vi "cn8202temp_controller.vi"(2 "?":bool, 3 "actions":cluster{bool, bool, bool, bool, bool}, 4 "Holdback (deg C)":dbl min=0.0 max=55.5 format="%.1f", 5 "Ramp Soak Recipe":string[][](table), 6 "Recycle #":dbl min=0.0 max=100.0, 7 "Setpoint (deg C)":dbl max=1200.0 format="%.3f") -> (0 "Current Recipe \nSetpoint (deg C)":dbl format="%.3f", 1 "Thermometer":dbl(slide) scale=0.0..1000.0 scale format="%.2f")   [LabVIEW 2012]
uses:
  <vilib>/Instr/_visa.llb/VISA Configure Serial Port (Instr).vi
panel:
  # "Omega CN8202 Control Program"
  # "Ramp/Soak Parameters"
  # "(0-55.5, 0=off)"
  # "(0-99, 100 = continuous)"
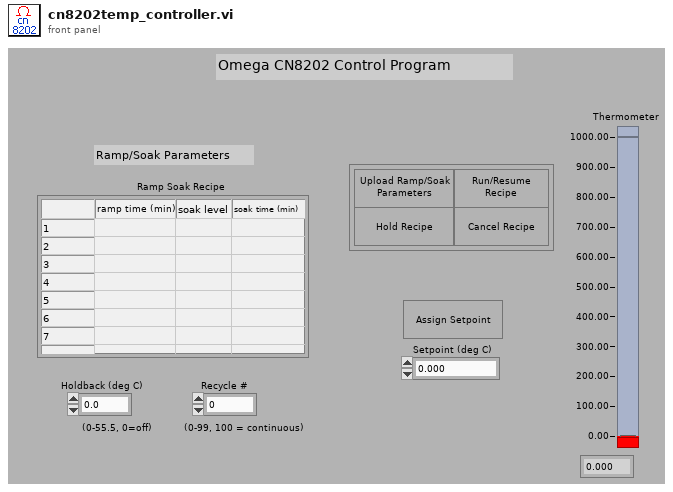
[diagram p1: front panel]
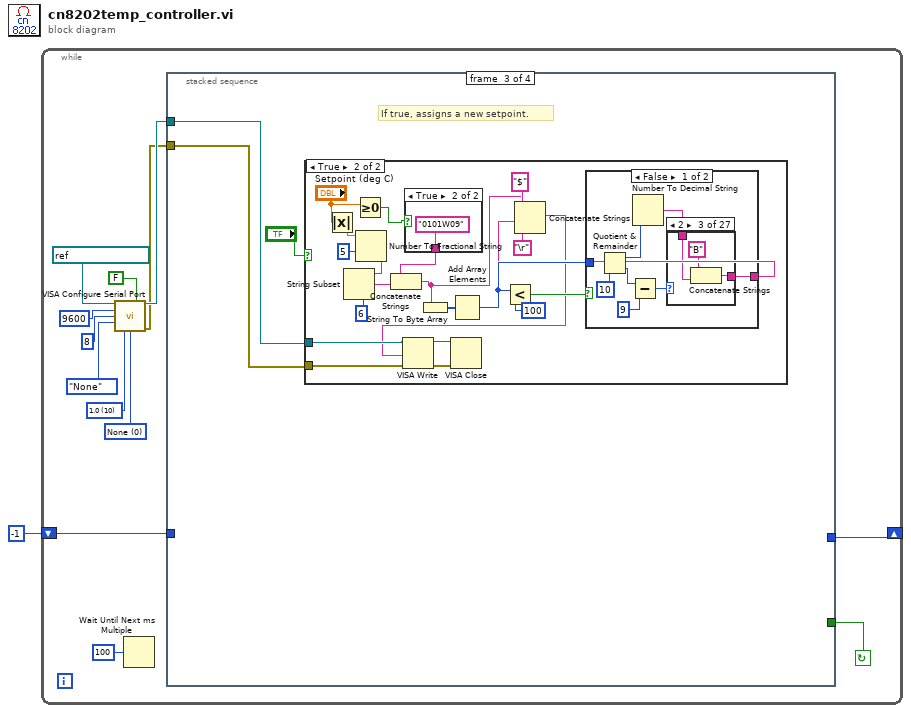
[diagram p0: block diagram]
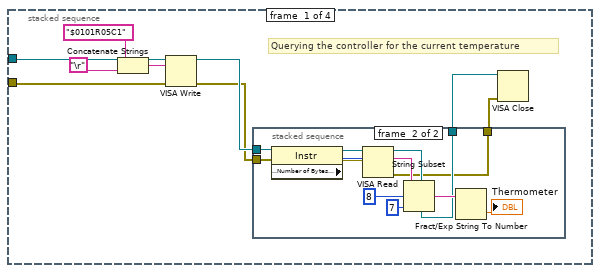
[diagram p2: hidden frame]
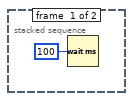
[diagram p3: hidden frame]
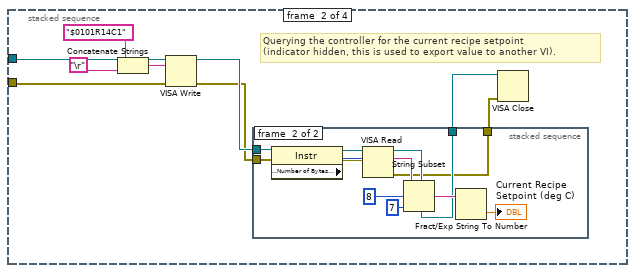
[diagram p4: hidden frame]
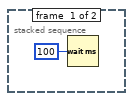
[diagram p5: hidden frame]
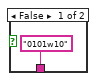
[diagram p7: hidden frame]
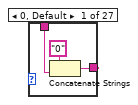
[diagram p8: hidden frame]
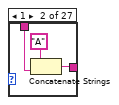
[diagram p9: hidden frame]
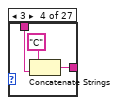
[diagram p10: hidden frame]
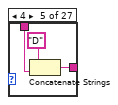
[diagram p11: hidden frame]
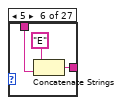
[diagram p12: hidden frame]
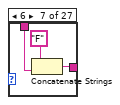
[diagram p13: hidden frame]
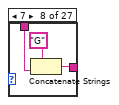
[diagram p14: hidden frame]
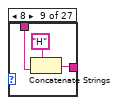
[diagram p15: hidden frame]
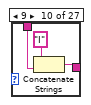
[diagram p16: hidden frame]
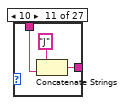
[diagram p17: hidden frame]
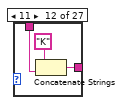
[diagram p18: hidden frame]
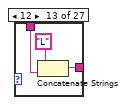
[diagram p19: hidden frame]
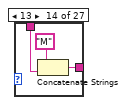
[diagram p20: hidden frame]
diagram:
  n1 = while {
    shift-right: [w2] -> _
    shift-left: -1 -> [w4]
    stop <- w3 continue-if-true
    w11 = u16 0 items=["None"=0, "XON/XOFF"=1, "RTS/CTS"=2, "DTR/DSR"=4] ("flow control (0:none)")
    w12 = u16 10 items=["1.0"=10, "1.5"=15, "2.0"=20] ("stop bits (10: 1 bit)")
    n2 = call-poly "VISA Configure Serial Port"("VISA resource name"=refnum<visa-resource-name> "ASRL1::INSTR", "Enable Termination\nChar (T)"=FALSE ("Enable Termination\nChar (T)"), "baud rate (9600)"=u32 9600, "data bits (8)"=u16 8, "parity (0:none)"=enum16{"None", "Odd", "Even", "Mark", "Space"}."None", "stop bits (10: 1 bit)"=w12, "flow control (0:none)"=w11) -> ("VISA resource name out"=w6:refnum<visa-resource-name>, "error out"=w5:errorcluster)  [unwired: 7 in]
    n3 = Wait Until Next ms Multiple(millisecond multiple=u32 100) -> ()  [unwired: 1 out]
    n4 = stacked-sequence {
      tunnel: w6 -> [w20 w42 w61 w180]
      tunnel: w5 -> [w19 w41 w60 w179]
      tunnel: w4 -> [_ _ _ w178]
      tunnel: [_ _ _ w177] -> w2
      tunnel: [_ _ _ w176] -> w3
      frame #0 {
        # "Querying the controller for the current temperature"
        n5 = Concatenate Strings("$0101R05C1", "\r") -> (w23:string)
        n6 = VISA Write(VISA resource name=w20, write buffer=w23, error in (no error)=w19) -> (VISA resource name out=w18:refnum<visa-resource-name>, error out=w17:errorcluster)  [unwired: 1 out]
        n7 = stacked-sequence {
          tunnel: w18 -> [_ w28]
          tunnel: w17 -> [_ w27]
          tunnel: [_ w26] -> w16
          tunnel: [_ w25] -> w15
          frame #0 {
            n8 = Wait (ms)(milliseconds to wait=u32 100) -> ()  [unwired: 1 out]
          }
          frame #1 {
            n9 = property class="Instr"(reference=w28, error in=w27) -> (reference out=w36:refnum<visa-resource-name>, error out=w34:errorcluster, "Serial Settings:Number of Bytes at Serial Port"=w35:u32)
            n10 = VISA Read(VISA resource name=w36, byte count=w35, error in (no error)=w34) -> (VISA resource name out=w26:refnum<visa-resource-name>, read buffer=w32:string, error out=w25:errorcluster)  [unwired: 1 out]
            n11 = String Subset(string=w32, offset (0)=8, length (rest)=7 ("length (rest)")) -> (substring=w31:string)
            n12 = Fract/Exp String To Number(string=w31) -> (number=→"Thermometer":dbl)  [unwired: 3 in, 1 out]
          }
        }
        n13 = VISA Close(VISA resource name=w16, error in (no error)=w15) -> ()  [unwired: 1 out]
      }
      frame #1 {
        # "Querying the controller for the current recipe setpoint\n(indicator hidden, this is used to export value to another VI)."
        n14 = Concatenate Strings("$0101R14C1", "\r") -> (w45:string)
        n15 = VISA Write(VISA resource name=w42, write buffer=w45, error in (no error)=w41) -> (VISA resource name out=w40:refnum<visa-resource-name>, error out=w39:errorcluster)  [unwired: 1 out]
        n16 = stacked-sequence {
          tunnel: w40 -> [_ w51]
          tunnel: w39 -> [_ w50]
          tunnel: [_ w49] -> w38
          tunnel: [_ w48] -> w37
          frame #0 {
            n17 = Wait (ms)(milliseconds to wait=u32 100) -> ()  [unwired: 1 out]
          }
          frame #1 {
            n18 = property class="Instr"(reference=w51, error in=w50) -> (reference out=w58:refnum<visa-resource-name>, error out=w56:errorcluster, "Serial Settings:Number of Bytes at Serial Port"=w57:u32)
            n19 = VISA Read(VISA resource name=w58, byte count=w57, error in (no error)=w56) -> (VISA resource name out=w49:refnum<visa-resource-name>, read buffer=w54:string, error out=w48:errorcluster)  [unwired: 1 out]
            n20 = String Subset(string=w54, offset (0)=8, length (rest)=7 ("length (rest)")) -> (substring=w53:string)
            n21 = Fract/Exp String To Number(string=w53) -> (number=→"Current Recipe \nSetpoint (deg C)":dbl)  [unwired: 3 in, 1 out]
          }
        }
        n22 = VISA Close(VISA resource name=w38, error in (no error)=w37) -> ()  [unwired: 1 out]
      }
      frame #2 {
        # "If true, assigns a new setpoint."
        n23 = case shown="True" "?" {
          tunnel: w61 -> [_ w66]
          tunnel: w60 -> [_ w65]
          frame False {
          }
          frame True {
            n24 = Absolute Value(x="Setpoint (deg C)") -> (abs(x)=w71:dbl)
            n25 = Greater Or Equal To 0?(x="Setpoint (deg C)") -> (x >= 0?=w72:bool)
            n26 = Number To Fractional String(number=w71, width (-)=i16 5) -> (F-format string=w76:string)  [unwired: 2 in]
            n27 = String Subset(string=w76, length (rest)=6 ("length (rest)")) -> (substring=w73:string)  [unwired: 1 in]
            n28 = case shown="True" w72 {
              tunnel: ["0101w10" "0101W09"] -> w69
              frame False {
              }
              frame True {
              }
            }
            n29 = Concatenate Strings(w69, w73) -> (w62:string)
            n30 = String To Byte Array(string=w62) -> (unsigned byte array=w82:u8[])
            n31 = Add Array Elements(numeric array=w82) -> (sum=w74:u8)
            n32 = Less?(x=w74, y=u8 100) -> (x < y?=w80:bool)
            n33 = case shown="False" w80 {
              tunnel: w74 -> [w88 w175]
              tunnel: [w87 w174] -> w70
              frame False {
                n34 = Quotient & Remainder(x=w88, y=u8 10) -> (x-y*floor(x/y)=w86:u8, floor(x/y)=w89:u8)
                n35 = Subtract(x=w89, y=u8 9) -> (x-y=w91:u8)
                n36 = Number To Decimal String(number=w86) -> (decimal integer string=w92:string)  [unwired: 1 in]
                n37 = case shown="2" w91 {
                  tunnel: w92 -> [w94 w97 w100 w103 w106 w109 w112 w115 w118 w121 w124 w127 w130 w133 w136 w139 w142 w145 w148 w151 w154 w157 w160 w163 w166 w169 w172]
                  tunnel: [w93 w96 w99 w102 w105 w108 w111 w114 w117 w120 w123 w126 w129 w132 w135 w138 w141 w144 w147 w150 w153 w156 w159 w162 w165 w168 w171] -> w87
                  frame 0, Default {
                    n38 = Concatenate Strings("0", w94) -> (w93:string)
                  }
                  frame 1 {
                    n39 = Concatenate Strings("A", w97) -> (w96:string)
                  }
                  frame 2 {
                    n40 = Concatenate Strings("B", w100) -> (w99:string)
                  }
                  frame 3 {
                    n41 = Concatenate Strings("C", w103) -> (w102:string)
                  }
                  frame 4 {
                    n42 = Concatenate Strings("D", w106) -> (w105:string)
                  }
                  frame 5 {
                    n43 = Concatenate Strings("E", w109) -> (w108:string)
                  }
                  frame 6 {
                    n44 = Concatenate Strings("F", w112) -> (w111:string)
                  }
                  frame 7 {
                    n45 = Concatenate Strings("G", w115) -> (w114:string)
                  }
                  frame 8 {
                    n46 = Concatenate Strings("H", w118) -> (w117:string)
                  }
                  frame 9 {
                    n47 = Concatenate Strings("I", w121) -> (w120:string)
                  }
                  frame 10 {
                    n48 = Concatenate Strings("J", w124) -> (w123:string)
                  }
                  frame 11 {
                    n49 = Concatenate Strings("K", w127) -> (w126:string)
                  }
                  frame 12 {
                    n50 = Concatenate Strings("L", w130) -> (w129:string)
                  }
                  frame 13 {
                    n51 = Concatenate Strings("M", w133) -> (w132:string)
                  }
                  frame 14 {
                    n52 = Concatenate Strings("N", w136) -> (w135:string)
                  }
                  frame 15 {
                    n53 = Concatenate Strings("O", w139) -> (w138:string)
                  }
                  frame 16 {
                    n54 = Concatenate Strings("P", w142) -> (w141:string)
                  }
                  frame 17 {
                    n55 = Concatenate Strings("Q", w145) -> (w144:string)
                  }
                  frame 18 {
                    n56 = Concatenate Strings("R", w148) -> (w147:string)
                  }
                  frame 19 {
                    n57 = Concatenate Strings("S", w151) -> (w150:string)
                  }
                  frame 20 {
                    n58 = Concatenate Strings("T", w154) -> (w153:string)
                  }
                  frame 21 {
                    n59 = Concatenate Strings("U", w157) -> (w156:string)
                  }
                  frame 22 {
                    n60 = Concatenate Strings("V", w160) -> (w159:string)
                  }
                  frame 23 {
                    n61 = Concatenate Strings("W", w163) -> (w162:string)
                  }
                  frame 24 {
                    n62 = Concatenate Strings("X", w166) -> (w165:string)
                  }
                  frame 25 {
                    n63 = Concatenate Strings("Y", w169) -> (w168:string)
                  }
                  frame 26 {
                    n64 = Concatenate Strings("Z", w172) -> (w171:string)
                  }
                }
              }
              frame True {
                n65 = Number To Decimal String(number=w175) -> (decimal integer string=w174:string)  [unwired: 1 in]
              }
            }
            n66 = Concatenate Strings("$", w62, w70, "\r") -> (w64:string)
            n67 = VISA Write(VISA resource name=w66, write buffer=w64, error in (no error)=w65) -> (VISA resource name out=w68:refnum<visa-resource-name>, error out=w67:errorcluster)  [unwired: 1 out]
            n68 = VISA Close(VISA resource name=w68, error in (no error)=w67) -> ()  [unwired: 1 out]
          }
        }
      }
      frame #3 {
        n69 = case shown="-1, Default" w178 {
          tunnel: [w181 -1 -1 -1 -1 -1 ("index of element")] -> w177
          tunnel: w180 -> [_ w188 w3077 w3085 w3092 _]
          tunnel: w179 -> [_ w187 w3076 w3086 w3091 _]
          tunnel: [TRUE TRUE TRUE TRUE TRUE FALSE] -> w176
          frame -1, Default {
            # "Check to see which button was pressed\nthen determine which \"state\" to execute next"
            # "No Button Pressed"
            n70 = Cluster To Array(cluster="actions") -> (array=w184:bool[])
            n71 = Search 1D Array(1D array=w184, element=TRUE) -> (index of element=w181:i32)  [unwired: 1 in]
          }
          frame 0 {
            # "Upload Parameters Button Pressed"
            n72 = stacked-sequence {
              tunnel: w188 -> [w192 w2850]
              tunnel: w187 -> [w191 w2849]
              frame #0 {
                # "Set Holdback Button Pressed"
                n73 = for {
                  N: 8 -> [_]
                  tunnel: "Ramp Soak Recipe" -> [w222]
                  tunnel: w192 -> [w201]
                  tunnel: w191 -> [w200]
                  i -> [w221]
                  n74 = Index Array(array=w222, index (row)=w221) -> (element=w220:string[])  [unwired: 1 in]
                  n75 = Index Array(array=w220, index=0) -> (element=w216:string)
                  n76 = Index Array(array=w220, index=1) -> (element=w203:string)
                  n77 = Index Array(array=w220, index=2) -> (element=w204:string)
                  n78 = Fract/Exp String To Number(string=w216) -> (number=w213:dbl)  [unwired: 3 in, 1 out]
                  n79 = Fract/Exp String To Number(string=w203) -> (number=w197:dbl)  [unwired: 3 in, 1 out]
                  n80 = Fract/Exp String To Number(string=w204) -> (number=w206:dbl)  [unwired: 3 in, 1 out]
                  n81 = Absolute Value(x=w197) -> (abs(x)=w194:dbl)
                  n82 = Number To Fractional String(number=w213, width (-)=i16 5) -> (F-format string=w212:string)  [unwired: 2 in]
                  n83 = Number To Fractional String(number=w194, width (-)=i16 5) -> (F-format string=w209:string)  [unwired: 2 in]
                  n84 = Number To Fractional String(number=w206, width (-)=i16 5) -> (F-format string=w205:string)  [unwired: 2 in]
                  n85 = String Subset(string=w212, length (rest)=6 ("length (rest)")) -> (substring=w202:string)  [unwired: 1 in]
                  n86 = String Subset(string=w209, length (rest)=6 ("length (rest)")) -> (substring=w199:string)  [unwired: 1 in]
                  n87 = String Subset(string=w205, length (rest)=6 ("length (rest)")) -> (substring=w198:string)  [unwired: 1 in]
                  n88 = Greater Or Equal To 0?(x=w197) -> (x >= 0?=w196:bool)
                  n89 = case shown="True" w196 {
                    tunnel: ["0101w" "0101W"] -> w195
                    frame False {
                    }
                    frame True {
                    }
                  }
                  n90 = case shown="0, Default" w221 {
                    tunnel: w202 -> [w225 w558 w886 w1214 w1542 w1870 w2198 w2526]
                    tunnel: w201 -> [w229 w556 w884 w1212 w1540 w1868 w2196 w2524]
                    tunnel: w200 -> [w228 w555 w883 w1211 w1539 w1867 w2195 w2523]
                    tunnel: w199 -> [w230 w557 w885 w1213 w1541 w1869 w2197 w2525]
                    tunnel: w198 -> [w227 w554 w882 w1210 w1538 w1866 w2194 w2522]
                    tunnel: w195 -> [w226 w553 w881 w1209 w1537 w1865 w2193 w2521]
                    frame 0, Default {
                      n91 = stacked-sequence {
                        tunnel: w225 -> [w239 _ _]
                        tunnel: w230 -> [_ w340 _]
                        tunnel: w229 -> [w233 w344 w450]
                        tunnel: w228 -> [w232 w343 w449]
                        tunnel: w227 -> [_ _ w447]
                        tunnel: w226 -> [_ w338 _]
                        frame #0 {
                          n92 = Wait Until Next ms Multiple(millisecond multiple=u32 300) -> ()  [unwired: 1 out]
                          n93 = Concatenate Strings("0101W42", w239) -> (w241:string)
                          n94 = String To Byte Array(string=w241) -> (unsigned byte array=w245:u8[])
                          n95 = Add Array Elements(numeric array=w245) -> (sum=w236:u8)
                          n96 = Less?(x=w236, y=u8 100) -> (x < y?=w238:bool)
                          n97 = case shown="False" w238 {
                            tunnel: w236 -> [w250 w337]
                            tunnel: [w249 w336] -> w237
                            frame False {
                              n98 = Quotient & Remainder(x=w250, y=u8 10) -> (x-y*floor(x/y)=w248:u8, floor(x/y)=w251:u8)
                              n99 = Subtract(x=w251, y=u8 9) -> (x-y=w253:u8)
                              n100 = Number To Decimal String(number=w248) -> (decimal integer string=w254:string)  [unwired: 1 in]
                              n101 = case shown="6" w253 {
                                tunnel: w254 -> [w256 w259 w262 w265 w268 w271 w274 w277 w280 w283 w286 w289 w292 w295 w298 w301 w304 w307 w310 w313 w316 w319 w322 w325 w328 w331 w334]
                                tunnel: [w255 w258 w261 w264 w267 w270 w273 w276 w279 w282 w285 w288 w291 w294 w297 w300 w303 w306 w309 w312 w315 w318 w321 w324 w327 w330 w333] -> w249
                                frame 0, Default {
                                n102 = Concatenate Strings("0", w256) -> (w255:string)
                                }
                                frame 1 {
                                n103 = Concatenate Strings("A", w259) -> (w258:string)
                                }
                                frame 2 {
                                n104 = Concatenate Strings("B", w262) -> (w261:string)
                                }
                                frame 3 {
                                n105 = Concatenate Strings("C", w265) -> (w264:string)
                                }
                                frame 4 {
                                n106 = Concatenate Strings("D", w268) -> (w267:string)
                                }
                                frame 5 {
                                n107 = Concatenate Strings("E", w271) -> (w270:string)
                                }
                                frame 6 {
                                n108 = Concatenate Strings("F", w274) -> (w273:string)
                                }
                                frame 7 {
                                n109 = Concatenate Strings("G", w277) -> (w276:string)
                                }
                                frame 8 {
                                n110 = Concatenate Strings("H", w280) -> (w279:string)
                                }
                                frame 9 {
                                n111 = Concatenate Strings("I", w283) -> (w282:string)
                                }
                                frame 10 {
                                n112 = Concatenate Strings("J", w286) -> (w285:string)
                                }
                                frame 11 {
                                n113 = Concatenate Strings("K", w289) -> (w288:string)
                                }
                                frame 12 {
                                n114 = Concatenate Strings("L", w292) -> (w291:string)
                                }
                                frame 13 {
                                n115 = Concatenate Strings("M", w295) -> (w294:string)
                                }
                                frame 14 {
                                n116 = Concatenate Strings("N", w298) -> (w297:string)
                                }
                                frame 15 {
                                n117 = Concatenate Strings("O", w301) -> (w300:string)
                                }
                                frame 16 {
                                n118 = Concatenate Strings("P", w304) -> (w303:string)
                                }
                                frame 17 {
                                n119 = Concatenate Strings("Q", w307) -> (w306:string)
                                }
                                frame 18 {
                                n120 = Concatenate Strings("R", w310) -> (w309:string)
                                }
                                frame 19 {
                                n121 = Concatenate Strings("S", w313) -> (w312:string)
                                }
                                frame 20 {
                                n122 = Concatenate Strings("T", w316) -> (w315:string)
                                }
                                frame 21 {
                                n123 = Concatenate Strings("U", w319) -> (w318:string)
                                }
                                frame 22 {
                                n124 = Concatenate Strings("V", w322) -> (w321:string)
                                }
                                frame 23 {
                                n125 = Concatenate Strings("W", w325) -> (w324:string)
                                }
                                frame 24 {
                                n126 = Concatenate Strings("X", w328) -> (w327:string)
                                }
                                frame 25 {
                                n127 = Concatenate Strings("Y", w331) -> (w330:string)
                                }
                                frame 26 {
                                n128 = Concatenate Strings("Z", w334) -> (w333:string)
                                }
                              }
                            }
                            frame True {
                              n129 = Number To Decimal String(number=w337) -> (decimal integer string=w336:string)  [unwired: 1 in]
                            }
                          }
                          n130 = Concatenate Strings("$", w241, w237, "\r") -> (w246:string)
                          n131 = VISA Write(VISA resource name=w233, write buffer=w246, error in (no error)=w232) -> (VISA resource name out=w235:refnum<visa-resource-name>, error out=w234:errorcluster)  [unwired: 1 out]
                          n132 = VISA Close(VISA resource name=w235, error in (no error)=w234) -> ()  [unwired: 1 out]
                        }
                        frame #1 {
                          n133 = Wait Until Next ms Multiple(millisecond multiple=u32 300) -> ()  [unwired: 1 out]
                          n134 = Concatenate Strings(w338, "58", w340) -> (w350:string)
                          n135 = String To Byte Array(string=w350) -> (unsigned byte array=w354:u8[])
                          n136 = Add Array Elements(numeric array=w354) -> (sum=w347:u8)
                          n137 = Less?(x=w347, y=u8 100) -> (x < y?=w349:bool)
                          n138 = case shown="False" w349 {
                            tunnel: w347 -> [w358 w445]
                            tunnel: [w357 w444] -> w348
                            frame False {
                              n139 = Quotient & Remainder(x=w358, y=u8 10) -> (x-y*floor(x/y)=w356:u8, floor(x/y)=w359:u8)
                              n140 = Subtract(x=w359, y=u8 9) -> (x-y=w361:u8)
                              n141 = Number To Decimal String(number=w356) -> (decimal integer string=w362:string)  [unwired: 1 in]
                              n142 = case shown="7" w361 {
                                tunnel: w362 -> [w364 w367 w370 w373 w376 w379 w382 w385 w388 w391 w394 w397 w400 w403 w406 w409 w412 w415 w418 w421 w424 w427 w430 w433 w436 w439 w442]
                                tunnel: [w363 w366 w369 w372 w375 w378 w381 w384 w387 w390 w393 w396 w399 w402 w405 w408 w411 w414 w417 w420 w423 w426 w429 w432 w435 w438 w441] -> w357
                                frame 0, Default {
                                n143 = Concatenate Strings("0", w364) -> (w363:string)
                                }
                                frame 1 {
                                n144 = Concatenate Strings("A", w367) -> (w366:string)
                                }
                                frame 2 {
                                n145 = Concatenate Strings("B", w370) -> (w369:string)
                                }
                                frame 3 {
                                n146 = Concatenate Strings("C", w373) -> (w372:string)
                                }
                                frame 4 {
                                n147 = Concatenate Strings("D", w376) -> (w375:string)
                                }
                                frame 5 {
                                n148 = Concatenate Strings("E", w379) -> (w378:string)
                                }
                                frame 6 {
                                n149 = Concatenate Strings("F", w382) -> (w381:string)
                                }
                                frame 7 {
                                n150 = Concatenate Strings("G", w385) -> (w384:string)
                                }
                                frame 8 {
                                n151 = Concatenate Strings("H", w388) -> (w387:string)
                                }
                                frame 9 {
                                n152 = Concatenate Strings("I", w391) -> (w390:string)
                                }
                                frame 10 {
                                n153 = Concatenate Strings("J", w394) -> (w393:string)
                                }
                                frame 11 {
                                n154 = Concatenate Strings("K", w397) -> (w396:string)
                                }
                                frame 12 {
                                n155 = Concatenate Strings("L", w400) -> (w399:string)
                                }
                                frame 13 {
                                n156 = Concatenate Strings("M", w403) -> (w402:string)
                                }
                                frame 14 {
                                n157 = Concatenate Strings("N", w406) -> (w405:string)
                                }
                                frame 15 {
                                n158 = Concatenate Strings("O", w409) -> (w408:string)
                                }
                                frame 16 {
                                n159 = Concatenate Strings("P", w412) -> (w411:string)
                                }
                                frame 17 {
                                n160 = Concatenate Strings("Q", w415) -> (w414:string)
                                }
                                frame 18 {
                                n161 = Concatenate Strings("R", w418) -> (w417:string)
                                }
                                frame 19 {
                                n162 = Concatenate Strings("S", w421) -> (w420:string)
                                }
                                frame 20 {
                                n163 = Concatenate Strings("T", w424) -> (w423:string)
                                }
                                frame 21 {
                                n164 = Concatenate Strings("U", w427) -> (w426:string)
                                }
                                frame 22 {
                                n165 = Concatenate Strings("V", w430) -> (w429:string)
                                }
                                frame 23 {
                                n166 = Concatenate Strings("W", w433) -> (w432:string)
                                }
                                frame 24 {
                                n167 = Concatenate Strings("X", w436) -> (w435:string)
                                }
                                frame 25 {
                                n168 = Concatenate Strings("Y", w439) -> (w438:string)
                                }
                                frame 26 {
                                n169 = Concatenate Strings("Z", w442) -> (w441:string)
                                }
                              }
                            }
                            frame True {
                              n170 = Number To Decimal String(number=w445) -> (decimal integer string=w444:string)  [unwired: 1 in]
                            }
                          }
                          n171 = Concatenate Strings("$", w350, w348, "\r") -> (w342:string)
                          n172 = VISA Write(VISA resource name=w344, write buffer=w342, error in (no error)=w343) -> (VISA resource name out=w346:refnum<visa-resource-name>, error out=w345:errorcluster)  [unwired: 1 out]
                          n173 = VISA Close(VISA resource name=w346, error in (no error)=w345) -> ()  [unwired: 1 out]
                        }
                        frame #2 {
                          n174 = Wait Until Next ms Multiple(millisecond multiple=u32 300) -> ()  [unwired: 1 out]
                          n175 = Concatenate Strings("0101W66", w447) -> (w457:string)
                          n176 = String To Byte Array(string=w457) -> (unsigned byte array=w461:u8[])
                          n177 = Add Array Elements(numeric array=w461) -> (sum=w453:u8)
                          n178 = Less?(x=w453, y=u8 100) -> (x < y?=w455:bool)
                          n179 = case shown="False" w455 {
                            tunnel: w453 -> [w465 w552]
                            tunnel: [w464 w551] -> w454
                            frame False {
                              n180 = Quotient & Remainder(x=w465, y=u8 10) -> (x-y*floor(x/y)=w463:u8, floor(x/y)=w466:u8)
                              n181 = Subtract(x=w466, y=u8 9) -> (x-y=w468:u8)
                              n182 = Number To Decimal String(number=w463) -> (decimal integer string=w469:string)  [unwired: 1 in]
                              n183 = case shown="7" w468 {
                                tunnel: w469 -> [w471 w474 w477 w480 w483 w486 w489 w492 w495 w498 w501 w504 w507 w510 w513 w516 w519 w522 w525 w528 w531 w534 w537 w540 w543 w546 w549]
                                tunnel: [w470 w473 w476 w479 w482 w485 w488 w491 w494 w497 w500 w503 w506 w509 w512 w515 w518 w521 w524 w527 w530 w533 w536 w539 w542 w545 w548] -> w464
                                frame 0, Default {
                                n184 = Concatenate Strings("0", w471) -> (w470:string)
                                }
                                frame 1 {
                                n185 = Concatenate Strings("A", w474) -> (w473:string)
                                }
                                frame 2 {
                                n186 = Concatenate Strings("B", w477) -> (w476:string)
                                }
                                frame 3 {
                                n187 = Concatenate Strings("C", w480) -> (w479:string)
                                }
                                frame 4 {
                                n188 = Concatenate Strings("D", w483) -> (w482:string)
                                }
                                frame 5 {
                                n189 = Concatenate Strings("E", w486) -> (w485:string)
                                }
                                frame 6 {
                                n190 = Concatenate Strings("F", w489) -> (w488:string)
                                }
                                frame 7 {
                                n191 = Concatenate Strings("G", w492) -> (w491:string)
                                }
                                frame 8 {
                                n192 = Concatenate Strings("H", w495) -> (w494:string)
                                }
                                frame 9 {
                                n193 = Concatenate Strings("I", w498) -> (w497:string)
                                }
                                frame 10 {
                                n194 = Concatenate Strings("J", w501) -> (w500:string)
                                }
                                frame 11 {
                                n195 = Concatenate Strings("K", w504) -> (w503:string)
                                }
                                frame 12 {
                                n196 = Concatenate Strings("L", w507) -> (w506:string)
                                }
                                frame 13 {
                                n197 = Concatenate Strings("M", w510) -> (w509:string)
                                }
                                frame 14 {
                                n198 = Concatenate Strings("N", w513) -> (w512:string)
                                }
                                frame 15 {
                                n199 = Concatenate Strings("O", w516) -> (w515:string)
                                }
                                frame 16 {
                                n200 = Concatenate Strings("P", w519) -> (w518:string)
                                }
                                frame 17 {
                                n201 = Concatenate Strings("Q", w522) -> (w521:string)
                                }
                                frame 18 {
                                n202 = Concatenate Strings("R", w525) -> (w524:string)
                                }
                                frame 19 {
                                n203 = Concatenate Strings("S", w528) -> (w527:string)
                                }
                                frame 20 {
                                n204 = Concatenate Strings("T", w531) -> (w530:string)
                                }
                                frame 21 {
                                n205 = Concatenate Strings("U", w534) -> (w533:string)
                                }
                                frame 22 {
                                n206 = Concatenate Strings("V", w537) -> (w536:string)
                                }
                                frame 23 {
                                n207 = Concatenate Strings("W", w540) -> (w539:string)
                                }
                                frame 24 {
                                n208 = Concatenate Strings("X", w543) -> (w542:string)
                                }
                                frame 25 {
                                n209 = Concatenate Strings("Y", w546) -> (w545:string)
                                }
                                frame 26 {
                                n210 = Concatenate Strings("Z", w549) -> (w548:string)
                                }
                              }
                            }
                            frame True {
                              n211 = Number To Decimal String(number=w552) -> (decimal integer string=w551:string)  [unwired: 1 in]
                            }
                          }
                          n212 = Concatenate Strings("$", w457, w454, "\r") -> (w448:string)
                          n213 = VISA Write(VISA resource name=w450, write buffer=w448, error in (no error)=w449) -> (VISA resource name out=w452:refnum<visa-resource-name>, error out=w451:errorcluster)  [unwired: 1 out]
                          n214 = VISA Close(VISA resource name=w452, error in (no error)=w451) -> ()  [unwired: 1 out]
                        }
                      }
                    }
                    frame 1 {
                      n215 = stacked-sequence {
                        tunnel: w558 -> [w567 _ _]
                        tunnel: w557 -> [_ w668 _]
                        tunnel: w556 -> [w561 w672 w778]
                        tunnel: w555 -> [w560 w671 w777]
                        tunnel: w554 -> [_ _ w775]
                        tunnel: w553 -> [_ w666 _]
                        frame #0 {
                          n216 = Wait Until Next ms Multiple(millisecond multiple=u32 300) -> ()  [unwired: 1 out]
                          n217 = Concatenate Strings("0101W43", w567) -> (w569:string)
                          n218 = String To Byte Array(string=w569) -> (unsigned byte array=w573:u8[])
                          n219 = Add Array Elements(numeric array=w573) -> (sum=w564:u8)
                          n220 = Less?(x=w564, y=u8 100) -> (x < y?=w566:bool)
                          n221 = case shown="False" w566 {
                            tunnel: w564 -> [w578 w665]
                            tunnel: [w577 w664] -> w565
                            frame False {
                              n222 = Quotient & Remainder(x=w578, y=u8 10) -> (x-y*floor(x/y)=w576:u8, floor(x/y)=w579:u8)
                              n223 = Subtract(x=w579, y=u8 9) -> (x-y=w581:u8)
                              n224 = Number To Decimal String(number=w576) -> (decimal integer string=w582:string)  [unwired: 1 in]
                              n225 = case shown="8" w581 {
                                tunnel: w582 -> [w584 w587 w590 w593 w596 w599 w602 w605 w608 w611 w614 w617 w620 w623 w626 w629 w632 w635 w638 w641 w644 w647 w650 w653 w656 w659 w662]
                                tunnel: [w583 w586 w589 w592 w595 w598 w601 w604 w607 w610 w613 w616 w619 w622 w625 w628 w631 w634 w637 w640 w643 w646 w649 w652 w655 w658 w661] -> w577
                                frame 0, Default {
                                n226 = Concatenate Strings("0", w584) -> (w583:string)
                                }
                                frame 1 {
                                n227 = Concatenate Strings("A", w587) -> (w586:string)
                                }
                                frame 2 {
                                n228 = Concatenate Strings("B", w590) -> (w589:string)
                                }
                                frame 3 {
                                n229 = Concatenate Strings("C", w593) -> (w592:string)
                                }
                                frame 4 {
                                n230 = Concatenate Strings("D", w596) -> (w595:string)
                                }
                                frame 5 {
                                n231 = Concatenate Strings("E", w599) -> (w598:string)
                                }
                                frame 6 {
                                n232 = Concatenate Strings("F", w602) -> (w601:string)
                                }
                                frame 7 {
                                n233 = Concatenate Strings("G", w605) -> (w604:string)
                                }
                                frame 8 {
                                n234 = Concatenate Strings("H", w608) -> (w607:string)
                                }
                                frame 9 {
                                n235 = Concatenate Strings("I", w611) -> (w610:string)
                                }
                                frame 10 {
                                n236 = Concatenate Strings("J", w614) -> (w613:string)
                                }
                                frame 11 {
                                n237 = Concatenate Strings("K", w617) -> (w616:string)
                                }
                                frame 12 {
                                n238 = Concatenate Strings("L", w620) -> (w619:string)
                                }
                                frame 13 {
                                n239 = Concatenate Strings("M", w623) -> (w622:string)
                                }
                                frame 14 {
                                n240 = Concatenate Strings("N", w626) -> (w625:string)
                                }
                                frame 15 {
                                n241 = Concatenate Strings("O", w629) -> (w628:string)
                                }
                                frame 16 {
                                n242 = Concatenate Strings("P", w632) -> (w631:string)
                                }
                                frame 17 {
                                n243 = Concatenate Strings("Q", w635) -> (w634:string)
                                }
                                frame 18 {
                                n244 = Concatenate Strings("R", w638) -> (w637:string)
                                }
                                frame 19 {
                                n245 = Concatenate Strings("S", w641) -> (w640:string)
                                }
                                frame 20 {
                                n246 = Concatenate Strings("T", w644) -> (w643:string)
                                }
                                frame 21 {
                                n247 = Concatenate Strings("U", w647) -> (w646:string)
                                }
                                frame 22 {
                                n248 = Concatenate Strings("V", w650) -> (w649:string)
                                }
                                frame 23 {
                                n249 = Concatenate Strings("W", w653) -> (w652:string)
                                }
                                frame 24 {
                                n250 = Concatenate Strings("X", w656) -> (w655:string)
                                }
                                frame 25 {
                                n251 = Concatenate Strings("Y", w659) -> (w658:string)
                                }
                                frame 26 {
                                n252 = Concatenate Strings("Z", w662) -> (w661:string)
                                }
                              }
                            }
                            frame True {
                              n253 = Number To Decimal String(number=w665) -> (decimal integer string=w664:string)  [unwired: 1 in]
                            }
                          }
                          n254 = Concatenate Strings("$", w569, w565, "\r") -> (w574:string)
                          n255 = VISA Write(VISA resource name=w561, write buffer=w574, error in (no error)=w560) -> (VISA resource name out=w563:refnum<visa-resource-name>, error out=w562:errorcluster)  [unwired: 1 out]
                          n256 = VISA Close(VISA resource name=w563, error in (no error)=w562) -> ()  [unwired: 1 out]
                        }
                        frame #1 {
                          n257 = Wait Until Next ms Multiple(millisecond multiple=u32 300) -> ()  [unwired: 1 out]
                          n258 = Concatenate Strings(w666, "59", w668) -> (w678:string)
                          n259 = String To Byte Array(string=w678) -> (unsigned byte array=w682:u8[])
                          n260 = Add Array Elements(numeric array=w682) -> (sum=w675:u8)
                          n261 = Less?(x=w675, y=u8 100) -> (x < y?=w677:bool)
                          n262 = case shown="False" w677 {
                            tunnel: w675 -> [w686 w773]
                            tunnel: [w685 w772] -> w676
                            frame False {
                              n263 = Quotient & Remainder(x=w686, y=u8 10) -> (x-y*floor(x/y)=w684:u8, floor(x/y)=w687:u8)
                              n264 = Subtract(x=w687, y=u8 9) -> (x-y=w689:u8)
                              n265 = Number To Decimal String(number=w684) -> (decimal integer string=w690:string)  [unwired: 1 in]
                              n266 = case shown="10" w689 {
                                tunnel: w690 -> [w692 w695 w698 w701 w704 w707 w710 w713 w716 w719 w722 w725 w728 w731 w734 w737 w740 w743 w746 w749 w752 w755 w758 w761 w764 w767 w770]
                                tunnel: [w691 w694 w697 w700 w703 w706 w709 w712 w715 w718 w721 w724 w727 w730 w733 w736 w739 w742 w745 w748 w751 w754 w757 w760 w763 w766 w769] -> w685
                                frame 0, Default {
                                n267 = Concatenate Strings("0", w692) -> (w691:string)
                                }
                                frame 1 {
                                n268 = Concatenate Strings("A", w695) -> (w694:string)
                                }
                                frame 2 {
                                n269 = Concatenate Strings("B", w698) -> (w697:string)
                                }
                                frame 3 {
                                n270 = Concatenate Strings("C", w701) -> (w700:string)
                                }
                                frame 4 {
                                n271 = Concatenate Strings("D", w704) -> (w703:string)
                                }
                                frame 5 {
                                n272 = Concatenate Strings("E", w707) -> (w706:string)
                                }
                                frame 6 {
                                n273 = Concatenate Strings("F", w710) -> (w709:string)
                                }
                                frame 7 {
                                n274 = Concatenate Strings("G", w713) -> (w712:string)
                                }
                                frame 8 {
                                n275 = Concatenate Strings("H", w716) -> (w715:string)
                                }
                                frame 9 {
                                n276 = Concatenate Strings("I", w719) -> (w718:string)
                                }
                                frame 10 {
                                n277 = Concatenate Strings("J", w722) -> (w721:string)
                                }
                                frame 11 {
                                n278 = Concatenate Strings("K", w725) -> (w724:string)
                                }
                                frame 12 {
                                n279 = Concatenate Strings("L", w728) -> (w727:string)
                                }
                                frame 13 {
                                n280 = Concatenate Strings("M", w731) -> (w730:string)
                                }
                                frame 14 {
                                n281 = Concatenate Strings("N", w734) -> (w733:string)
                                }
                                frame 15 {
                                n282 = Concatenate Strings("O", w737) -> (w736:string)
                                }
                                frame 16 {
                                n283 = Concatenate Strings("P", w740) -> (w739:string)
                                }
                                frame 17 {
                                n284 = Concatenate Strings("Q", w743) -> (w742:string)
                                }
                                frame 18 {
                                n285 = Concatenate Strings("R", w746) -> (w745:string)
                                }
                                frame 19 {
                                n286 = Concatenate Strings("S", w749) -> (w748:string)
                                }
                                frame 20 {
                                n287 = Concatenate Strings("T", w752) -> (w751:string)
                                }
                                frame 21 {
                                n288 = Concatenate Strings("U", w755) -> (w754:string)
                                }
                                frame 22 {
                                n289 = Concatenate Strings("V", w758) -> (w757:string)
                                }
                                frame 23 {
                                n290 = Concatenate Strings("W", w761) -> (w760:string)
                                }
                                frame 24 {
                                n291 = Concatenate Strings("X", w764) -> (w763:string)
                                }
                                frame 25 {
                                n292 = Concatenate Strings("Y", w767) -> (w766:string)
                                }
                                frame 26 {
                                n293 = Concatenate Strings("Z", w770) -> (w769:string)
                                }
                              }
                            }
                            frame True {
                              n294 = Number To Decimal String(number=w773) -> (decimal integer string=w772:string)  [unwired: 1 in]
                            }
                          }
                          n295 = Concatenate Strings("$", w678, w676, "\r") -> (w670:string)
                          n296 = VISA Write(VISA resource name=w672, write buffer=w670, error in (no error)=w671) -> (VISA resource name out=w674:refnum<visa-resource-name>, error out=w673:errorcluster)  [unwired: 1 out]
                          n297 = VISA Close(VISA resource name=w674, error in (no error)=w673) -> ()  [unwired: 1 out]
                        }
                        frame #2 {
                          n298 = Wait Until Next ms Multiple(millisecond multiple=u32 300) -> ()  [unwired: 1 out]
                          n299 = Concatenate Strings("0101W67", w775) -> (w785:string)
                          n300 = String To Byte Array(string=w785) -> (unsigned byte array=w789:u8[])
                          n301 = Add Array Elements(numeric array=w789) -> (sum=w781:u8)
                          n302 = Less?(x=w781, y=u8 100) -> (x < y?=w783:bool)
                          n303 = case shown="False" w783 {
                            tunnel: w781 -> [w793 w880]
                            tunnel: [w792 w879] -> w782
                            frame False {
                              n304 = Quotient & Remainder(x=w793, y=u8 10) -> (x-y*floor(x/y)=w791:u8, floor(x/y)=w794:u8)
                              n305 = Subtract(x=w794, y=u8 9) -> (x-y=w796:u8)
                              n306 = Number To Decimal String(number=w791) -> (decimal integer string=w797:string)  [unwired: 1 in]
                              n307 = case shown="8" w796 {
                                tunnel: w797 -> [w799 w802 w805 w808 w811 w814 w817 w820 w823 w826 w829 w832 w835 w838 w841 w844 w847 w850 w853 w856 w859 w862 w865 w868 w871 w874 w877]
                                tunnel: [w798 w801 w804 w807 w810 w813 w816 w819 w822 w825 w828 w831 w834 w837 w840 w843 w846 w849 w852 w855 w858 w861 w864 w867 w870 w873 w876] -> w792
                                frame 0, Default {
                                n308 = Concatenate Strings("0", w799) -> (w798:string)
                                }
                                frame 1 {
                                n309 = Concatenate Strings("A", w802) -> (w801:string)
                                }
                                frame 2 {
                                n310 = Concatenate Strings("B", w805) -> (w804:string)
                                }
                                frame 3 {
                                n311 = Concatenate Strings("C", w808) -> (w807:string)
                                }
                                frame 4 {
                                n312 = Concatenate Strings("D", w811) -> (w810:string)
                                }
                                frame 5 {
                                n313 = Concatenate Strings("E", w814) -> (w813:string)
                                }
                                frame 6 {
                                n314 = Concatenate Strings("F", w817) -> (w816:string)
                                }
                                frame 7 {
                                n315 = Concatenate Strings("G", w820) -> (w819:string)
                                }
                                frame 8 {
                                n316 = Concatenate Strings("H", w823) -> (w822:string)
                                }
                                frame 9 {
                                n317 = Concatenate Strings("I", w826) -> (w825:string)
                                }
                                frame 10 {
                                n318 = Concatenate Strings("J", w829) -> (w828:string)
                                }
                                frame 11 {
                                n319 = Concatenate Strings("K", w832) -> (w831:string)
                                }
                                frame 12 {
                                n320 = Concatenate Strings("L", w835) -> (w834:string)
                                }
                                frame 13 {
                                n321 = Concatenate Strings("M", w838) -> (w837:string)
                                }
                                frame 14 {
                                n322 = Concatenate Strings("N", w841) -> (w840:string)
                                }
                                frame 15 {
                                n323 = Concatenate Strings("O", w844) -> (w843:string)
                                }
                                frame 16 {
                                n324 = Concatenate Strings("P", w847) -> (w846:string)
                                }
                                frame 17 {
                                n325 = Concatenate Strings("Q", w850) -> (w849:string)
                                }
                                frame 18 {
                                n326 = Concatenate Strings("R", w853) -> (w852:string)
                                }
                                frame 19 {
                                n327 = Concatenate Strings("S", w856) -> (w855:string)
                                }
                                frame 20 {
                                n328 = Concatenate Strings("T", w859) -> (w858:string)
                                }
                                frame 21 {
                                n329 = Concatenate Strings("U", w862) -> (w861:string)
                                }
                                frame 22 {
                                n330 = Concatenate Strings("V", w865) -> (w864:string)
                                }
                                frame 23 {
                                n331 = Concatenate Strings("W", w868) -> (w867:string)
                                }
                                frame 24 {
                                n332 = Concatenate Strings("X", w871) -> (w870:string)
                                }
                                frame 25 {
                                n333 = Concatenate Strings("Y", w874) -> (w873:string)
                                }
                                frame 26 {
                                n334 = Concatenate Strings("Z", w877) -> (w876:string)
                                }
                              }
                            }
                            frame True {
                              n335 = Number To Decimal String(number=w880) -> (decimal integer string=w879:string)  [unwired: 1 in]
                            }
                          }
                          n336 = Concatenate Strings("$", w785, w782, "\r") -> (w776:string)
                          n337 = VISA Write(VISA resource name=w778, write buffer=w776, error in (no error)=w777) -> (VISA resource name out=w780:refnum<visa-resource-name>, error out=w779:errorcluster)  [unwired: 1 out]
                          n338 = VISA Close(VISA resource name=w780, error in (no error)=w779) -> ()  [unwired: 1 out]
                        }
                      }
                    }
                    frame 2 {
                      n339 = stacked-sequence {
                        tunnel: w886 -> [w895 _ _]
                        tunnel: w885 -> [_ w996 _]
                        tunnel: w884 -> [w889 w1000 w1106]
                        tunnel: w883 -> [w888 w999 w1105]
                        tunnel: w882 -> [_ _ w1103]
                        tunnel: w881 -> [_ w994 _]
                        frame #0 {
                          n340 = Wait Until Next ms Multiple(millisecond multiple=u32 300) -> ()  [unwired: 1 out]
                          n341 = Concatenate Strings("0101W44", w895) -> (w897:string)
                          n342 = String To Byte Array(string=w897) -> (unsigned byte array=w901:u8[])
                          n343 = Add Array Elements(numeric array=w901) -> (sum=w892:u8)
                          n344 = Less?(x=w892, y=u8 100) -> (x < y?=w894:bool)
                          n345 = case shown="False" w894 {
                            tunnel: w892 -> [w906 w993]
                            tunnel: [w905 w992] -> w893
                            frame False {
                              n346 = Quotient & Remainder(x=w906, y=u8 10) -> (x-y*floor(x/y)=w904:u8, floor(x/y)=w907:u8)
                              n347 = Subtract(x=w907, y=u8 9) -> (x-y=w909:u8)
                              n348 = Number To Decimal String(number=w904) -> (decimal integer string=w910:string)  [unwired: 1 in]
                              n349 = case shown="6" w909 {
                                tunnel: w910 -> [w912 w915 w918 w921 w924 w927 w930 w933 w936 w939 w942 w945 w948 w951 w954 w957 w960 w963 w966 w969 w972 w975 w978 w981 w984 w987 w990]
                                tunnel: [w911 w914 w917 w920 w923 w926 w929 w932 w935 w938 w941 w944 w947 w950 w953 w956 w959 w962 w965 w968 w971 w974 w977 w980 w983 w986 w989] -> w905
                                frame 0, Default {
                                n350 = Concatenate Strings("0", w912) -> (w911:string)
                                }
                                frame 1 {
                                n351 = Concatenate Strings("A", w915) -> (w914:string)
                                }
                                frame 2 {
                                n352 = Concatenate Strings("B", w918) -> (w917:string)
                                }
                                frame 3 {
                                n353 = Concatenate Strings("C", w921) -> (w920:string)
                                }
                                frame 4 {
                                n354 = Concatenate Strings("D", w924) -> (w923:string)
                                }
                                frame 5 {
                                n355 = Concatenate Strings("E", w927) -> (w926:string)
                                }
                                frame 6 {
                                n356 = Concatenate Strings("F", w930) -> (w929:string)
                                }
                                frame 7 {
                                n357 = Concatenate Strings("G", w933) -> (w932:string)
                                }
                                frame 8 {
                                n358 = Concatenate Strings("H", w936) -> (w935:string)
                                }
                                frame 9 {
                                n359 = Concatenate Strings("I", w939) -> (w938:string)
                                }
                                frame 10 {
                                n360 = Concatenate Strings("J", w942) -> (w941:string)
                                }
                                frame 11 {
                                n361 = Concatenate Strings("K", w945) -> (w944:string)
                                }
                                frame 12 {
                                n362 = Concatenate Strings("L", w948) -> (w947:string)
                                }
                                frame 13 {
                                n363 = Concatenate Strings("M", w951) -> (w950:string)
                                }
                                frame 14 {
                                n364 = Concatenate Strings("N", w954) -> (w953:string)
                                }
                                frame 15 {
                                n365 = Concatenate Strings("O", w957) -> (w956:string)
                                }
                                frame 16 {
                                n366 = Concatenate Strings("P", w960) -> (w959:string)
                                }
                                frame 17 {
                                n367 = Concatenate Strings("Q", w963) -> (w962:string)
                                }
                                frame 18 {
                                n368 = Concatenate Strings("R", w966) -> (w965:string)
                                }
                                frame 19 {
                                n369 = Concatenate Strings("S", w969) -> (w968:string)
                                }
                                frame 20 {
                                n370 = Concatenate Strings("T", w972) -> (w971:string)
                                }
                                frame 21 {
                                n371 = Concatenate Strings("U", w975) -> (w974:string)
                                }
                                frame 22 {
                                n372 = Concatenate Strings("V", w978) -> (w977:string)
                                }
                                frame 23 {
                                n373 = Concatenate Strings("W", w981) -> (w980:string)
                                }
                                frame 24 {
                                n374 = Concatenate Strings("X", w984) -> (w983:string)
                                }
                                frame 25 {
                                n375 = Concatenate Strings("Y", w987) -> (w986:string)
                                }
                                frame 26 {
                                n376 = Concatenate Strings("Z", w990) -> (w989:string)
                                }
                              }
                            }
                            frame True {
                              n377 = Number To Decimal String(number=w993) -> (decimal integer string=w992:string)  [unwired: 1 in]
                            }
                          }
                          n378 = Concatenate Strings("$", w897, w893, "\r") -> (w902:string)
                          n379 = VISA Write(VISA resource name=w889, write buffer=w902, error in (no error)=w888) -> (VISA resource name out=w891:refnum<visa-resource-name>, error out=w890:errorcluster)  [unwired: 1 out]
                          n380 = VISA Close(VISA resource name=w891, error in (no error)=w890) -> ()  [unwired: 1 out]
                        }
                        frame #1 {
                          n381 = Wait Until Next ms Multiple(millisecond multiple=u32 300) -> ()  [unwired: 1 out]
                          n382 = Concatenate Strings(w994, "60", w996) -> (w1006:string)
                          n383 = String To Byte Array(string=w1006) -> (unsigned byte array=w1010:u8[])
                          n384 = Add Array Elements(numeric array=w1010) -> (sum=w1003:u8)
                          n385 = Less?(x=w1003, y=u8 100) -> (x < y?=w1005:bool)
                          n386 = case shown="False" w1005 {
                            tunnel: w1003 -> [w1014 w1101]
                            tunnel: [w1013 w1100] -> w1004
                            frame False {
                              n387 = Quotient & Remainder(x=w1014, y=u8 10) -> (x-y*floor(x/y)=w1012:u8, floor(x/y)=w1015:u8)
                              n388 = Subtract(x=w1015, y=u8 9) -> (x-y=w1017:u8)
                              n389 = Number To Decimal String(number=w1012) -> (decimal integer string=w1018:string)  [unwired: 1 in]
                              n390 = case shown="11" w1017 {
                                tunnel: w1018 -> [w1020 w1023 w1026 w1029 w1032 w1035 w1038 w1041 w1044 w1047 w1050 w1053 w1056 w1059 w1062 w1065 w1068 w1071 w1074 w1077 w1080 w1083 w1086 w1089 w1092 w1095 w1098]
                                tunnel: [w1019 w1022 w1025 w1028 w1031 w1034 w1037 w1040 w1043 w1046 w1049 w1052 w1055 w1058 w1061 w1064 w1067 w1070 w1073 w1076 w1079 w1082 w1085 w1088 w1091 w1094 w1097] -> w1013
                                frame 0, Default {
                                n391 = Concatenate Strings("0", w1020) -> (w1019:string)
                                }
                                frame 1 {
                                n392 = Concatenate Strings("A", w1023) -> (w1022:string)
                                }
                                frame 2 {
                                n393 = Concatenate Strings("B", w1026) -> (w1025:string)
                                }
                                frame 3 {
                                n394 = Concatenate Strings("C", w1029) -> (w1028:string)
                                }
                                frame 4 {
                                n395 = Concatenate Strings("D", w1032) -> (w1031:string)
                                }
                                frame 5 {
                                n396 = Concatenate Strings("E", w1035) -> (w1034:string)
                                }
                                frame 6 {
                                n397 = Concatenate Strings("F", w1038) -> (w1037:string)
                                }
                                frame 7 {
                                n398 = Concatenate Strings("G", w1041) -> (w1040:string)
                                }
                                frame 8 {
                                n399 = Concatenate Strings("H", w1044) -> (w1043:string)
                                }
                                frame 9 {
                                n400 = Concatenate Strings("I", w1047) -> (w1046:string)
                                }
                                frame 10 {
                                n401 = Concatenate Strings("J", w1050) -> (w1049:string)
                                }
                                frame 11 {
                                n402 = Concatenate Strings("K", w1053) -> (w1052:string)
                                }
                                frame 12 {
                                n403 = Concatenate Strings("L", w1056) -> (w1055:string)
                                }
                                frame 13 {
                                n404 = Concatenate Strings("M", w1059) -> (w1058:string)
                                }
                                frame 14 {
                                n405 = Concatenate Strings("N", w1062) -> (w1061:string)
                                }
                                frame 15 {
                                n406 = Concatenate Strings("O", w1065) -> (w1064:string)
                                }
                                frame 16 {
                                n407 = Concatenate Strings("P", w1068) -> (w1067:string)
                                }
                                frame 17 {
                                n408 = Concatenate Strings("Q", w1071) -> (w1070:string)
                                }
                                frame 18 {
                                n409 = Concatenate Strings("R", w1074) -> (w1073:string)
                                }
                                frame 19 {
                                n410 = Concatenate Strings("S", w1077) -> (w1076:string)
                                }
                                frame 20 {
                                n411 = Concatenate Strings("T", w1080) -> (w1079:string)
                                }
                                frame 21 {
                                n412 = Concatenate Strings("U", w1083) -> (w1082:string)
                                }
                                frame 22 {
                                n413 = Concatenate Strings("V", w1086) -> (w1085:string)
                                }
                                frame 23 {
                                n414 = Concatenate Strings("W", w1089) -> (w1088:string)
                                }
                                frame 24 {
                                n415 = Concatenate Strings("X", w1092) -> (w1091:string)
                                }
                                frame 25 {
                                n416 = Concatenate Strings("Y", w1095) -> (w1094:string)
                                }
                                frame 26 {
                                n417 = Concatenate Strings("Z", w1098) -> (w1097:string)
                                }
                              }
                            }
                            frame True {
                              n418 = Number To Decimal String(number=w1101) -> (decimal integer string=w1100:string)  [unwired: 1 in]
                            }
                          }
                          n419 = Concatenate Strings("$", w1006, w1004, "\r") -> (w998:string)
                          n420 = VISA Write(VISA resource name=w1000, write buffer=w998, error in (no error)=w999) -> (VISA resource name out=w1002:refnum<visa-resource-name>, error out=w1001:errorcluster)  [unwired: 1 out]
                          n421 = VISA Close(VISA resource name=w1002, error in (no error)=w1001) -> ()  [unwired: 1 out]
                        }
                        frame #2 {
                          n422 = Wait Until Next ms Multiple(millisecond multiple=u32 300) -> ()  [unwired: 1 out]
                          n423 = Concatenate Strings("0101W68", w1103) -> (w1113:string)
                          n424 = String To Byte Array(string=w1113) -> (unsigned byte array=w1117:u8[])
                          n425 = Add Array Elements(numeric array=w1117) -> (sum=w1109:u8)
                          n426 = Less?(x=w1109, y=u8 100) -> (x < y?=w1111:bool)
                          n427 = case shown="False" w1111 {
                            tunnel: w1109 -> [w1121 w1208]
                            tunnel: [w1120 w1207] -> w1110
                            frame False {
                              n428 = Quotient & Remainder(x=w1121, y=u8 10) -> (x-y*floor(x/y)=w1119:u8, floor(x/y)=w1122:u8)
                              n429 = Subtract(x=w1122, y=u8 9) -> (x-y=w1124:u8)
                              n430 = Number To Decimal String(number=w1119) -> (decimal integer string=w1125:string)  [unwired: 1 in]
                              n431 = case shown="7" w1124 {
                                tunnel: w1125 -> [w1127 w1130 w1133 w1136 w1139 w1142 w1145 w1148 w1151 w1154 w1157 w1160 w1163 w1166 w1169 w1172 w1175 w1178 w1181 w1184 w1187 w1190 w1193 w1196 w1199 w1202 w1205]
                                tunnel: [w1126 w1129 w1132 w1135 w1138 w1141 w1144 w1147 w1150 w1153 w1156 w1159 w1162 w1165 w1168 w1171 w1174 w1177 w1180 w1183 w1186 w1189 w1192 w1195 w1198 w1201 w1204] -> w1120
                                frame 0, Default {
                                n432 = Concatenate Strings("0", w1127) -> (w1126:string)
                                }
                                frame 1 {
                                n433 = Concatenate Strings("A", w1130) -> (w1129:string)
                                }
                                frame 2 {
                                n434 = Concatenate Strings("B", w1133) -> (w1132:string)
                                }
                                frame 3 {
                                n435 = Concatenate Strings("C", w1136) -> (w1135:string)
                                }
                                frame 4 {
                                n436 = Concatenate Strings("D", w1139) -> (w1138:string)
                                }
                                frame 5 {
                                n437 = Concatenate Strings("E", w1142) -> (w1141:string)
                                }
                                frame 6 {
                                n438 = Concatenate Strings("F", w1145) -> (w1144:string)
                                }
                                frame 7 {
                                n439 = Concatenate Strings("G", w1148) -> (w1147:string)
                                }
                                frame 8 {
                                n440 = Concatenate Strings("H", w1151) -> (w1150:string)
                                }
                                frame 9 {
                                n441 = Concatenate Strings("I", w1154) -> (w1153:string)
                                }
                                frame 10 {
                                n442 = Concatenate Strings("J", w1157) -> (w1156:string)
                                }
                                frame 11 {
                                n443 = Concatenate Strings("K", w1160) -> (w1159:string)
                                }
                                frame 12 {
                                n444 = Concatenate Strings("L", w1163) -> (w1162:string)
                                }
                                frame 13 {
                                n445 = Concatenate Strings("M", w1166) -> (w1165:string)
                                }
                                frame 14 {
                                n446 = Concatenate Strings("N", w1169) -> (w1168:string)
                                }
                                frame 15 {
                                n447 = Concatenate Strings("O", w1172) -> (w1171:string)
                                }
                                frame 16 {
                                n448 = Concatenate Strings("P", w1175) -> (w1174:string)
                                }
                                frame 17 {
                                n449 = Concatenate Strings("Q", w1178) -> (w1177:string)
                                }
                                frame 18 {
                                n450 = Concatenate Strings("R", w1181) -> (w1180:string)
                                }
                                frame 19 {
                                n451 = Concatenate Strings("S", w1184) -> (w1183:string)
                                }
                                frame 20 {
                                n452 = Concatenate Strings("T", w1187) -> (w1186:string)
                                }
                                frame 21 {
                                n453 = Concatenate Strings("U", w1190) -> (w1189:string)
                                }
                                frame 22 {
                                n454 = Concatenate Strings("V", w1193) -> (w1192:string)
                                }
                                frame 23 {
                                n455 = Concatenate Strings("W", w1196) -> (w1195:string)
                                }
                                frame 24 {
                                n456 = Concatenate Strings("X", w1199) -> (w1198:string)
                                }
                                frame 25 {
                                n457 = Concatenate Strings("Y", w1202) -> (w1201:string)
                                }
                                frame 26 {
                                n458 = Concatenate Strings("Z", w1205) -> (w1204:string)
                                }
                              }
                            }
                            frame True {
                              n459 = Number To Decimal String(number=w1208) -> (decimal integer string=w1207:string)  [unwired: 1 in]
                            }
                          }
                          n460 = Concatenate Strings("$", w1113, w1110, "\r") -> (w1104:string)
                          n461 = VISA Write(VISA resource name=w1106, write buffer=w1104, error in (no error)=w1105) -> (VISA resource name out=w1108:refnum<visa-resource-name>, error out=w1107:errorcluster)  [unwired: 1 out]
                          n462 = VISA Close(VISA resource name=w1108, error in (no error)=w1107) -> ()  [unwired: 1 out]
                        }
                      }
                    }
                    frame 3 {
                      n463 = stacked-sequence {
                        tunnel: w1214 -> [w1223 _ _]
                        tunnel: w1213 -> [_ w1324 _]
                        tunnel: w1212 -> [w1217 w1328 w1434]
                        tunnel: w1211 -> [w1216 w1327 w1433]
                        tunnel: w1210 -> [_ _ w1431]
                        tunnel: w1209 -> [_ w1322 _]
                        frame #0 {
                          n464 = Wait Until Next ms Multiple(millisecond multiple=u32 300) -> ()  [unwired: 1 out]
                          n465 = Concatenate Strings("0101W45", w1223) -> (w1225:string)
                          n466 = String To Byte Array(string=w1225) -> (unsigned byte array=w1229:u8[])
                          n467 = Add Array Elements(numeric array=w1229) -> (sum=w1220:u8)
                          n468 = Less?(x=w1220, y=u8 100) -> (x < y?=w1222:bool)
                          n469 = case shown="False" w1222 {
                            tunnel: w1220 -> [w1234 w1321]
                            tunnel: [w1233 w1320] -> w1221
                            frame False {
                              n470 = Quotient & Remainder(x=w1234, y=u8 10) -> (x-y*floor(x/y)=w1232:u8, floor(x/y)=w1235:u8)
                              n471 = Subtract(x=w1235, y=u8 9) -> (x-y=w1237:u8)
                              n472 = Number To Decimal String(number=w1232) -> (decimal integer string=w1238:string)  [unwired: 1 in]
                              n473 = case shown="7" w1237 {
                                tunnel: w1238 -> [w1240 w1243 w1246 w1249 w1252 w1255 w1258 w1261 w1264 w1267 w1270 w1273 w1276 w1279 w1282 w1285 w1288 w1291 w1294 w1297 w1300 w1303 w1306 w1309 w1312 w1315 w1318]
                                tunnel: [w1239 w1242 w1245 w1248 w1251 w1254 w1257 w1260 w1263 w1266 w1269 w1272 w1275 w1278 w1281 w1284 w1287 w1290 w1293 w1296 w1299 w1302 w1305 w1308 w1311 w1314 w1317] -> w1233
                                frame 0, Default {
                                n474 = Concatenate Strings("0", w1240) -> (w1239:string)
                                }
                                frame 1 {
                                n475 = Concatenate Strings("A", w1243) -> (w1242:string)
                                }
                                frame 2 {
                                n476 = Concatenate Strings("B", w1246) -> (w1245:string)
                                }
                                frame 3 {
                                n477 = Concatenate Strings("C", w1249) -> (w1248:string)
                                }
                                frame 4 {
                                n478 = Concatenate Strings("D", w1252) -> (w1251:string)
                                }
                                frame 5 {
                                n479 = Concatenate Strings("E", w1255) -> (w1254:string)
                                }
                                frame 6 {
                                n480 = Concatenate Strings("F", w1258) -> (w1257:string)
                                }
                                frame 7 {
                                n481 = Concatenate Strings("G", w1261) -> (w1260:string)
                                }
                                frame 8 {
                                n482 = Concatenate Strings("H", w1264) -> (w1263:string)
                                }
                                frame 9 {
                                n483 = Concatenate Strings("I", w1267) -> (w1266:string)
                                }
                                frame 10 {
                                n484 = Concatenate Strings("J", w1270) -> (w1269:string)
                                }
                                frame 11 {
                                n485 = Concatenate Strings("K", w1273) -> (w1272:string)
                                }
                                frame 12 {
                                n486 = Concatenate Strings("L", w1276) -> (w1275:string)
                                }
                                frame 13 {
                                n487 = Concatenate Strings("M", w1279) -> (w1278:string)
                                }
                                frame 14 {
                                n488 = Concatenate Strings("N", w1282) -> (w1281:string)
                                }
                                frame 15 {
                                n489 = Concatenate Strings("O", w1285) -> (w1284:string)
                                }
                                frame 16 {
                                n490 = Concatenate Strings("P", w1288) -> (w1287:string)
                                }
                                frame 17 {
                                n491 = Concatenate Strings("Q", w1291) -> (w1290:string)
                                }
                                frame 18 {
                                n492 = Concatenate Strings("R", w1294) -> (w1293:string)
                                }
                                frame 19 {
                                n493 = Concatenate Strings("S", w1297) -> (w1296:string)
                                }
                                frame 20 {
                                n494 = Concatenate Strings("T", w1300) -> (w1299:string)
                                }
                                frame 21 {
                                n495 = Concatenate Strings("U", w1303) -> (w1302:string)
                                }
                                frame 22 {
                                n496 = Concatenate Strings("V", w1306) -> (w1305:string)
                                }
                                frame 23 {
                                n497 = Concatenate Strings("W", w1309) -> (w1308:string)
                                }
                                frame 24 {
                                n498 = Concatenate Strings("X", w1312) -> (w1311:string)
                                }
                                frame 25 {
                                n499 = Concatenate Strings("Y", w1315) -> (w1314:string)
                                }
                                frame 26 {
                                n500 = Concatenate Strings("Z", w1318) -> (w1317:string)
                                }
                              }
                            }
                            frame True {
                              n501 = Number To Decimal String(number=w1321) -> (decimal integer string=w1320:string)  [unwired: 1 in]
                            }
                          }
                          n502 = Concatenate Strings("$", w1225, w1221, "\r") -> (w1230:string)
                          n503 = VISA Write(VISA resource name=w1217, write buffer=w1230, error in (no error)=w1216) -> (VISA resource name out=w1219:refnum<visa-resource-name>, error out=w1218:errorcluster)  [unwired: 1 out]
                          n504 = VISA Close(VISA resource name=w1219, error in (no error)=w1218) -> ()  [unwired: 1 out]
                        }
                        frame #1 {
                          n505 = Wait Until Next ms Multiple(millisecond multiple=u32 300) -> ()  [unwired: 1 out]
                          n506 = Concatenate Strings(w1322, "61", w1324) -> (w1334:string)
                          n507 = String To Byte Array(string=w1334) -> (unsigned byte array=w1338:u8[])
                          n508 = Add Array Elements(numeric array=w1338) -> (sum=w1331:u8)
                          n509 = Less?(x=w1331, y=u8 100) -> (x < y?=w1333:bool)
                          n510 = case shown="False" w1333 {
                            tunnel: w1331 -> [w1342 w1429]
                            tunnel: [w1341 w1428] -> w1332
                            frame False {
                              n511 = Quotient & Remainder(x=w1342, y=u8 10) -> (x-y*floor(x/y)=w1340:u8, floor(x/y)=w1343:u8)
                              n512 = Subtract(x=w1343, y=u8 9) -> (x-y=w1345:u8)
                              n513 = Number To Decimal String(number=w1340) -> (decimal integer string=w1346:string)  [unwired: 1 in]
                              n514 = case shown="10" w1345 {
                                tunnel: w1346 -> [w1348 w1351 w1354 w1357 w1360 w1363 w1366 w1369 w1372 w1375 w1378 w1381 w1384 w1387 w1390 w1393 w1396 w1399 w1402 w1405 w1408 w1411 w1414 w1417 w1420 w1423 w1426]
                                tunnel: [w1347 w1350 w1353 w1356 w1359 w1362 w1365 w1368 w1371 w1374 w1377 w1380 w1383 w1386 w1389 w1392 w1395 w1398 w1401 w1404 w1407 w1410 w1413 w1416 w1419 w1422 w1425] -> w1341
                                frame 0, Default {
                                n515 = Concatenate Strings("0", w1348) -> (w1347:string)
                                }
                                frame 1 {
                                n516 = Concatenate Strings("A", w1351) -> (w1350:string)
                                }
                                frame 2 {
                                n517 = Concatenate Strings("B", w1354) -> (w1353:string)
                                }
                                frame 3 {
                                n518 = Concatenate Strings("C", w1357) -> (w1356:string)
                                }
                                frame 4 {
                                n519 = Concatenate Strings("D", w1360) -> (w1359:string)
                                }
                                frame 5 {
                                n520 = Concatenate Strings("E", w1363) -> (w1362:string)
                                }
                                frame 6 {
                                n521 = Concatenate Strings("F", w1366) -> (w1365:string)
                                }
                                frame 7 {
                                n522 = Concatenate Strings("G", w1369) -> (w1368:string)
                                }
                                frame 8 {
                                n523 = Concatenate Strings("H", w1372) -> (w1371:string)
                                }
                                frame 9 {
                                n524 = Concatenate Strings("I", w1375) -> (w1374:string)
                                }
                                frame 10 {
                                n525 = Concatenate Strings("J", w1378) -> (w1377:string)
                                }
                                frame 11 {
                                n526 = Concatenate Strings("K", w1381) -> (w1380:string)
                                }
                                frame 12 {
                                n527 = Concatenate Strings("L", w1384) -> (w1383:string)
                                }
                                frame 13 {
                                n528 = Concatenate Strings("M", w1387) -> (w1386:string)
                                }
                                frame 14 {
                                n529 = Concatenate Strings("N", w1390) -> (w1389:string)
                                }
                                frame 15 {
                                n530 = Concatenate Strings("O", w1393) -> (w1392:string)
                                }
                                frame 16 {
                                n531 = Concatenate Strings("P", w1396) -> (w1395:string)
                                }
                                frame 17 {
                                n532 = Concatenate Strings("Q", w1399) -> (w1398:string)
                                }
                                frame 18 {
                                n533 = Concatenate Strings("R", w1402) -> (w1401:string)
                                }
                                frame 19 {
                                n534 = Concatenate Strings("S", w1405) -> (w1404:string)
                                }
                                frame 20 {
                                n535 = Concatenate Strings("T", w1408) -> (w1407:string)
                                }
                                frame 21 {
                                n536 = Concatenate Strings("U", w1411) -> (w1410:string)
                                }
                                frame 22 {
                                n537 = Concatenate Strings("V", w1414) -> (w1413:string)
                                }
                                frame 23 {
                                n538 = Concatenate Strings("W", w1417) -> (w1416:string)
                                }
                                frame 24 {
                                n539 = Concatenate Strings("X", w1420) -> (w1419:string)
                                }
                                frame 25 {
                                n540 = Concatenate Strings("Y", w1423) -> (w1422:string)
                                }
                                frame 26 {
                                n541 = Concatenate Strings("Z", w1426) -> (w1425:string)
                                }
                              }
                            }
                            frame True {
                              n542 = Number To Decimal String(number=w1429) -> (decimal integer string=w1428:string)  [unwired: 1 in]
                            }
                          }
                          n543 = Concatenate Strings("$", w1334, w1332, "\r") -> (w1326:string)
                          n544 = VISA Write(VISA resource name=w1328, write buffer=w1326, error in (no error)=w1327) -> (VISA resource name out=w1330:refnum<visa-resource-name>, error out=w1329:errorcluster)  [unwired: 1 out]
                          n545 = VISA Close(VISA resource name=w1330, error in (no error)=w1329) -> ()  [unwired: 1 out]
                        }
                        frame #2 {
                          n546 = Wait Until Next ms Multiple(millisecond multiple=u32 300) -> ()  [unwired: 1 out]
                          n547 = Concatenate Strings("0101W69", w1431) -> (w1441:string)
                          n548 = String To Byte Array(string=w1441) -> (unsigned byte array=w1445:u8[])
                          n549 = Add Array Elements(numeric array=w1445) -> (sum=w1437:u8)
                          n550 = Less?(x=w1437, y=u8 100) -> (x < y?=w1439:bool)
                          n551 = case shown="False" w1439 {
                            tunnel: w1437 -> [w1449 w1536]
                            tunnel: [w1448 w1535] -> w1438
                            frame False {
                              n552 = Quotient & Remainder(x=w1449, y=u8 10) -> (x-y*floor(x/y)=w1447:u8, floor(x/y)=w1450:u8)
                              n553 = Subtract(x=w1450, y=u8 9) -> (x-y=w1452:u8)
                              n554 = Number To Decimal String(number=w1447) -> (decimal integer string=w1453:string)  [unwired: 1 in]
                              n555 = case shown="7" w1452 {
                                tunnel: w1453 -> [w1455 w1458 w1461 w1464 w1467 w1470 w1473 w1476 w1479 w1482 w1485 w1488 w1491 w1494 w1497 w1500 w1503 w1506 w1509 w1512 w1515 w1518 w1521 w1524 w1527 w1530 w1533]
                                tunnel: [w1454 w1457 w1460 w1463 w1466 w1469 w1472 w1475 w1478 w1481 w1484 w1487 w1490 w1493 w1496 w1499 w1502 w1505 w1508 w1511 w1514 w1517 w1520 w1523 w1526 w1529 w1532] -> w1448
                                frame 0, Default {
                                n556 = Concatenate Strings("0", w1455) -> (w1454:string)
                                }
                                frame 1 {
                                n557 = Concatenate Strings("A", w1458) -> (w1457:string)
                                }
                                frame 2 {
                                n558 = Concatenate Strings("B", w1461) -> (w1460:string)
                                }
                                frame 3 {
                                n559 = Concatenate Strings("C", w1464) -> (w1463:string)
                                }
                                frame 4 {
                                n560 = Concatenate Strings("D", w1467) -> (w1466:string)
                                }
                                frame 5 {
                                n561 = Concatenate Strings("E", w1470) -> (w1469:string)
                                }
                                frame 6 {
                                n562 = Concatenate Strings("F", w1473) -> (w1472:string)
                                }
                                frame 7 {
                                n563 = Concatenate Strings("G", w1476) -> (w1475:string)
                                }
                                frame 8 {
                                n564 = Concatenate Strings("H", w1479) -> (w1478:string)
                                }
                                frame 9 {
                                n565 = Concatenate Strings("I", w1482) -> (w1481:string)
                                }
                                frame 10 {
                                n566 = Concatenate Strings("J", w1485) -> (w1484:string)
                                }
                                frame 11 {
                                n567 = Concatenate Strings("K", w1488) -> (w1487:string)
                                }
                                frame 12 {
                                n568 = Concatenate Strings("L", w1491) -> (w1490:string)
                                }
                                frame 13 {
                                n569 = Concatenate Strings("M", w1494) -> (w1493:string)
                                }
                                frame 14 {
                                n570 = Concatenate Strings("N", w1497) -> (w1496:string)
                                }
                                frame 15 {
                                n571 = Concatenate Strings("O", w1500) -> (w1499:string)
                                }
                                frame 16 {
                                n572 = Concatenate Strings("P", w1503) -> (w1502:string)
                                }
                                frame 17 {
                                n573 = Concatenate Strings("Q", w1506) -> (w1505:string)
                                }
                                frame 18 {
                                n574 = Concatenate Strings("R", w1509) -> (w1508:string)
                                }
                                frame 19 {
                                n575 = Concatenate Strings("S", w1512) -> (w1511:string)
                                }
                                frame 20 {
                                n576 = Concatenate Strings("T", w1515) -> (w1514:string)
                                }
                                frame 21 {
                                n577 = Concatenate Strings("U", w1518) -> (w1517:string)
                                }
                                frame 22 {
                                n578 = Concatenate Strings("V", w1521) -> (w1520:string)
                                }
                                frame 23 {
                                n579 = Concatenate Strings("W", w1524) -> (w1523:string)
                                }
                                frame 24 {
                                n580 = Concatenate Strings("X", w1527) -> (w1526:string)
                                }
                                frame 25 {
                                n581 = Concatenate Strings("Y", w1530) -> (w1529:string)
                                }
                                frame 26 {
                                n582 = Concatenate Strings("Z", w1533) -> (w1532:string)
                                }
                              }
                            }
                            frame True {
                              n583 = Number To Decimal String(number=w1536) -> (decimal integer string=w1535:string)  [unwired: 1 in]
                            }
                          }
                          n584 = Concatenate Strings("$", w1441, w1438, "\r") -> (w1432:string)
                          n585 = VISA Write(VISA resource name=w1434, write buffer=w1432, error in (no error)=w1433) -> (VISA resource name out=w1436:refnum<visa-resource-name>, error out=w1435:errorcluster)  [unwired: 1 out]
                          n586 = VISA Close(VISA resource name=w1436, error in (no error)=w1435) -> ()  [unwired: 1 out]
                        }
                      }
                    }
                    frame 4 {
                      n587 = stacked-sequence {
                        tunnel: w1542 -> [w1551 _ _]
                        tunnel: w1541 -> [_ w1651 _]
                        tunnel: w1540 -> [w1545 w1656 w1762]
                        tunnel: w1539 -> [w1544 w1655 w1761]
                        tunnel: w1538 -> [_ _ w1759]
                        tunnel: w1537 -> [_ w1650 _]
                        frame #0 {
                          n588 = Wait Until Next ms Multiple(millisecond multiple=u32 300) -> ()  [unwired: 1 out]
                          n589 = Concatenate Strings("0101W46", w1551) -> (w1553:string)
                          n590 = String To Byte Array(string=w1553) -> (unsigned byte array=w1557:u8[])
                          n591 = Add Array Elements(numeric array=w1557) -> (sum=w1548:u8)
                          n592 = Less?(x=w1548, y=u8 100) -> (x < y?=w1550:bool)
                          n593 = case shown="False" w1550 {
                            tunnel: w1548 -> [w1562 w1649]
                            tunnel: [w1561 w1648] -> w1549
                            frame False {
                              n594 = Quotient & Remainder(x=w1562, y=u8 10) -> (x-y*floor(x/y)=w1560:u8, floor(x/y)=w1563:u8)
                              n595 = Subtract(x=w1563, y=u8 9) -> (x-y=w1565:u8)
                              n596 = Number To Decimal String(number=w1560) -> (decimal integer string=w1566:string)  [unwired: 1 in]
                              n597 = case shown="7" w1565 {
                                tunnel: w1566 -> [w1568 w1571 w1574 w1577 w1580 w1583 w1586 w1589 w1592 w1595 w1598 w1601 w1604 w1607 w1610 w1613 w1616 w1619 w1622 w1625 w1628 w1631 w1634 w1637 w1640 w1643 w1646]
                                tunnel: [w1567 w1570 w1573 w1576 w1579 w1582 w1585 w1588 w1591 w1594 w1597 w1600 w1603 w1606 w1609 w1612 w1615 w1618 w1621 w1624 w1627 w1630 w1633 w1636 w1639 w1642 w1645] -> w1561
                                frame 0, Default {
                                n598 = Concatenate Strings("0", w1568) -> (w1567:string)
                                }
                                frame 1 {
                                n599 = Concatenate Strings("A", w1571) -> (w1570:string)
                                }
                                frame 2 {
                                n600 = Concatenate Strings("B", w1574) -> (w1573:string)
                                }
                                frame 3 {
                                n601 = Concatenate Strings("C", w1577) -> (w1576:string)
                                }
                                frame 4 {
                                n602 = Concatenate Strings("D", w1580) -> (w1579:string)
                                }
                                frame 5 {
                                n603 = Concatenate Strings("E", w1583) -> (w1582:string)
                                }
                                frame 6 {
                                n604 = Concatenate Strings("F", w1586) -> (w1585:string)
                                }
                                frame 7 {
                                n605 = Concatenate Strings("G", w1589) -> (w1588:string)
                                }
                                frame 8 {
                                n606 = Concatenate Strings("H", w1592) -> (w1591:string)
                                }
                                frame 9 {
                                n607 = Concatenate Strings("I", w1595) -> (w1594:string)
                                }
                                frame 10 {
                                n608 = Concatenate Strings("J", w1598) -> (w1597:string)
                                }
                                frame 11 {
                                n609 = Concatenate Strings("K", w1601) -> (w1600:string)
                                }
                                frame 12 {
                                n610 = Concatenate Strings("L", w1604) -> (w1603:string)
                                }
                                frame 13 {
                                n611 = Concatenate Strings("M", w1607) -> (w1606:string)
                                }
                                frame 14 {
                                n612 = Concatenate Strings("N", w1610) -> (w1609:string)
                                }
                                frame 15 {
                                n613 = Concatenate Strings("O", w1613) -> (w1612:string)
                                }
                                frame 16 {
                                n614 = Concatenate Strings("P", w1616) -> (w1615:string)
                                }
                                frame 17 {
                                n615 = Concatenate Strings("Q", w1619) -> (w1618:string)
                                }
                                frame 18 {
                                n616 = Concatenate Strings("R", w1622) -> (w1621:string)
                                }
                                frame 19 {
                                n617 = Concatenate Strings("S", w1625) -> (w1624:string)
                                }
                                frame 20 {
                                n618 = Concatenate Strings("T", w1628) -> (w1627:string)
                                }
                                frame 21 {
                                n619 = Concatenate Strings("U", w1631) -> (w1630:string)
                                }
                                frame 22 {
                                n620 = Concatenate Strings("V", w1634) -> (w1633:string)
                                }
                                frame 23 {
                                n621 = Concatenate Strings("W", w1637) -> (w1636:string)
                                }
                                frame 24 {
                                n622 = Concatenate Strings("X", w1640) -> (w1639:string)
                                }
                                frame 25 {
                                n623 = Concatenate Strings("Y", w1643) -> (w1642:string)
                                }
                                frame 26 {
                                n624 = Concatenate Strings("Z", w1646) -> (w1645:string)
                                }
                              }
                            }
                            frame True {
                              n625 = Number To Decimal String(number=w1649) -> (decimal integer string=w1648:string)  [unwired: 1 in]
                            }
                          }
                          n626 = Concatenate Strings("$", w1553, w1549, "\r") -> (w1558:string)
                          n627 = VISA Write(VISA resource name=w1545, write buffer=w1558, error in (no error)=w1544) -> (VISA resource name out=w1547:refnum<visa-resource-name>, error out=w1546:errorcluster)  [unwired: 1 out]
                          n628 = VISA Close(VISA resource name=w1547, error in (no error)=w1546) -> ()  [unwired: 1 out]
                        }
                        frame #1 {
                          n629 = Wait Until Next ms Multiple(millisecond multiple=u32 300) -> ()  [unwired: 1 out]
                          n630 = Concatenate Strings(w1650, "62", w1651) -> (w1662:string)
                          n631 = String To Byte Array(string=w1662) -> (unsigned byte array=w1666:u8[])
                          n632 = Add Array Elements(numeric array=w1666) -> (sum=w1659:u8)
                          n633 = Less?(x=w1659, y=u8 100) -> (x < y?=w1661:bool)
                          n634 = case shown="False" w1661 {
                            tunnel: w1659 -> [w1670 w1757]
                            tunnel: [w1669 w1756] -> w1660
                            frame False {
                              n635 = Quotient & Remainder(x=w1670, y=u8 10) -> (x-y*floor(x/y)=w1668:u8, floor(x/y)=w1671:u8)
                              n636 = Subtract(x=w1671, y=u8 9) -> (x-y=w1673:u8)
                              n637 = Number To Decimal String(number=w1668) -> (decimal integer string=w1674:string)  [unwired: 1 in]
                              n638 = case shown="8" w1673 {
                                tunnel: w1674 -> [w1676 w1679 w1682 w1685 w1688 w1691 w1694 w1697 w1700 w1703 w1706 w1709 w1712 w1715 w1718 w1721 w1724 w1727 w1730 w1733 w1736 w1739 w1742 w1745 w1748 w1751 w1754]
                                tunnel: [w1675 w1678 w1681 w1684 w1687 w1690 w1693 w1696 w1699 w1702 w1705 w1708 w1711 w1714 w1717 w1720 w1723 w1726 w1729 w1732 w1735 w1738 w1741 w1744 w1747 w1750 w1753] -> w1669
                                frame 0, Default {
                                n639 = Concatenate Strings("0", w1676) -> (w1675:string)
                                }
                                frame 1 {
                                n640 = Concatenate Strings("A", w1679) -> (w1678:string)
                                }
                                frame 2 {
                                n641 = Concatenate Strings("B", w1682) -> (w1681:string)
                                }
                                frame 3 {
                                n642 = Concatenate Strings("C", w1685) -> (w1684:string)
                                }
                                frame 4 {
                                n643 = Concatenate Strings("D", w1688) -> (w1687:string)
                                }
                                frame 5 {
                                n644 = Concatenate Strings("E", w1691) -> (w1690:string)
                                }
                                frame 6 {
                                n645 = Concatenate Strings("F", w1694) -> (w1693:string)
                                }
                                frame 7 {
                                n646 = Concatenate Strings("G", w1697) -> (w1696:string)
                                }
                                frame 8 {
                                n647 = Concatenate Strings("H", w1700) -> (w1699:string)
                                }
                                frame 9 {
                                n648 = Concatenate Strings("I", w1703) -> (w1702:string)
                                }
                                frame 10 {
                                n649 = Concatenate Strings("J", w1706) -> (w1705:string)
                                }
                                frame 11 {
                                n650 = Concatenate Strings("K", w1709) -> (w1708:string)
                                }
                                frame 12 {
                                n651 = Concatenate Strings("L", w1712) -> (w1711:string)
                                }
                                frame 13 {
                                n652 = Concatenate Strings("M", w1715) -> (w1714:string)
                                }
                                frame 14 {
                                n653 = Concatenate Strings("N", w1718) -> (w1717:string)
                                }
                                frame 15 {
                                n654 = Concatenate Strings("O", w1721) -> (w1720:string)
                                }
                                frame 16 {
                                n655 = Concatenate Strings("P", w1724) -> (w1723:string)
                                }
                                frame 17 {
                                n656 = Concatenate Strings("Q", w1727) -> (w1726:string)
                                }
                                frame 18 {
                                n657 = Concatenate Strings("R", w1730) -> (w1729:string)
                                }
                                frame 19 {
                                n658 = Concatenate Strings("S", w1733) -> (w1732:string)
                                }
                                frame 20 {
                                n659 = Concatenate Strings("T", w1736) -> (w1735:string)
                                }
                                frame 21 {
                                n660 = Concatenate Strings("U", w1739) -> (w1738:string)
                                }
                                frame 22 {
                                n661 = Concatenate Strings("V", w1742) -> (w1741:string)
                                }
                                frame 23 {
                                n662 = Concatenate Strings("W", w1745) -> (w1744:string)
                                }
                                frame 24 {
                                n663 = Concatenate Strings("X", w1748) -> (w1747:string)
                                }
                                frame 25 {
                                n664 = Concatenate Strings("Y", w1751) -> (w1750:string)
                                }
                                frame 26 {
                                n665 = Concatenate Strings("Z", w1754) -> (w1753:string)
                                }
                              }
                            }
                            frame True {
                              n666 = Number To Decimal String(number=w1757) -> (decimal integer string=w1756:string)  [unwired: 1 in]
                            }
                          }
                          n667 = Concatenate Strings("$", w1662, w1660, "\r") -> (w1654:string)
                          n668 = VISA Write(VISA resource name=w1656, write buffer=w1654, error in (no error)=w1655) -> (VISA resource name out=w1658:refnum<visa-resource-name>, error out=w1657:errorcluster)  [unwired: 1 out]
                          n669 = VISA Close(VISA resource name=w1658, error in (no error)=w1657) -> ()  [unwired: 1 out]
                        }
                        frame #2 {
                          n670 = Wait Until Next ms Multiple(millisecond multiple=u32 300) -> ()  [unwired: 1 out]
                          n671 = Concatenate Strings("0101W70", w1759) -> (w1769:string)
                          n672 = String To Byte Array(string=w1769) -> (unsigned byte array=w1773:u8[])
                          n673 = Add Array Elements(numeric array=w1773) -> (sum=w1765:u8)
                          n674 = Less?(x=w1765, y=u8 100) -> (x < y?=w1767:bool)
                          n675 = case shown="False" w1767 {
                            tunnel: w1765 -> [w1777 w1864]
                            tunnel: [w1776 w1863] -> w1766
                            frame False {
                              n676 = Quotient & Remainder(x=w1777, y=u8 10) -> (x-y*floor(x/y)=w1775:u8, floor(x/y)=w1778:u8)
                              n677 = Subtract(x=w1778, y=u8 9) -> (x-y=w1780:u8)
                              n678 = Number To Decimal String(number=w1775) -> (decimal integer string=w1781:string)  [unwired: 1 in]
                              n679 = case shown="8" w1780 {
                                tunnel: w1781 -> [w1783 w1786 w1789 w1792 w1795 w1798 w1801 w1804 w1807 w1810 w1813 w1816 w1819 w1822 w1825 w1828 w1831 w1834 w1837 w1840 w1843 w1846 w1849 w1852 w1855 w1858 w1861]
                                tunnel: [w1782 w1785 w1788 w1791 w1794 w1797 w1800 w1803 w1806 w1809 w1812 w1815 w1818 w1821 w1824 w1827 w1830 w1833 w1836 w1839 w1842 w1845 w1848 w1851 w1854 w1857 w1860] -> w1776
                                frame 0, Default {
                                n680 = Concatenate Strings("0", w1783) -> (w1782:string)
                                }
                                frame 1 {
                                n681 = Concatenate Strings("A", w1786) -> (w1785:string)
                                }
                                frame 2 {
                                n682 = Concatenate Strings("B", w1789) -> (w1788:string)
                                }
                                frame 3 {
                                n683 = Concatenate Strings("C", w1792) -> (w1791:string)
                                }
                                frame 4 {
                                n684 = Concatenate Strings("D", w1795) -> (w1794:string)
                                }
                                frame 5 {
                                n685 = Concatenate Strings("E", w1798) -> (w1797:string)
                                }
                                frame 6 {
                                n686 = Concatenate Strings("F", w1801) -> (w1800:string)
                                }
                                frame 7 {
                                n687 = Concatenate Strings("G", w1804) -> (w1803:string)
                                }
                                frame 8 {
                                n688 = Concatenate Strings("H", w1807) -> (w1806:string)
                                }
                                frame 9 {
                                n689 = Concatenate Strings("I", w1810) -> (w1809:string)
                                }
                                frame 10 {
                                n690 = Concatenate Strings("J", w1813) -> (w1812:string)
                                }
                                frame 11 {
                                n691 = Concatenate Strings("K", w1816) -> (w1815:string)
                                }
                                frame 12 {
                                n692 = Concatenate Strings("L", w1819) -> (w1818:string)
                                }
                                frame 13 {
                                n693 = Concatenate Strings("M", w1822) -> (w1821:string)
                                }
                                frame 14 {
                                n694 = Concatenate Strings("N", w1825) -> (w1824:string)
                                }
                                frame 15 {
                                n695 = Concatenate Strings("O", w1828) -> (w1827:string)
                                }
                                frame 16 {
                                n696 = Concatenate Strings("P", w1831) -> (w1830:string)
                                }
                                frame 17 {
                                n697 = Concatenate Strings("Q", w1834) -> (w1833:string)
                                }
                                frame 18 {
                                n698 = Concatenate Strings("R", w1837) -> (w1836:string)
                                }
                                frame 19 {
                                n699 = Concatenate Strings("S", w1840) -> (w1839:string)
                                }
                                frame 20 {
                                n700 = Concatenate Strings("T", w1843) -> (w1842:string)
                                }
                                frame 21 {
                                n701 = Concatenate Strings("U", w1846) -> (w1845:string)
                                }
                                frame 22 {
                                n702 = Concatenate Strings("V", w1849) -> (w1848:string)
                                }
                                frame 23 {
                                n703 = Concatenate Strings("W", w1852) -> (w1851:string)
                                }
                                frame 24 {
                                n704 = Concatenate Strings("X", w1855) -> (w1854:string)
                                }
                                frame 25 {
                                n705 = Concatenate Strings("Y", w1858) -> (w1857:string)
                                }
                                frame 26 {
                                n706 = Concatenate Strings("Z", w1861) -> (w1860:string)
                                }
                              }
                            }
                            frame True {
                              n707 = Number To Decimal String(number=w1864) -> (decimal integer string=w1863:string)  [unwired: 1 in]
                            }
                          }
                          n708 = Concatenate Strings("$", w1769, w1766, "\r") -> (w1760:string)
                          n709 = VISA Write(VISA resource name=w1762, write buffer=w1760, error in (no error)=w1761) -> (VISA resource name out=w1764:refnum<visa-resource-name>, error out=w1763:errorcluster)  [unwired: 1 out]
                          n710 = VISA Close(VISA resource name=w1764, error in (no error)=w1763) -> ()  [unwired: 1 out]
                        }
                      }
                    }
                    frame 5 {
                      n711 = stacked-sequence {
                        tunnel: w1870 -> [w1879 _ _]
                        tunnel: w1869 -> [_ w1978 _]
                        tunnel: w1868 -> [w1873 w1984 w2090]
                        tunnel: w1867 -> [w1872 w1983 w2089]
                        tunnel: w1866 -> [_ _ w2087]
                        tunnel: w1865 -> [_ w1980 _]
                        frame #0 {
                          n712 = Wait Until Next ms Multiple(millisecond multiple=u32 300) -> ()  [unwired: 1 out]
                          n713 = Concatenate Strings("0101W47", w1879) -> (w1881:string)
                          n714 = String To Byte Array(string=w1881) -> (unsigned byte array=w1885:u8[])
                          n715 = Add Array Elements(numeric array=w1885) -> (sum=w1876:u8)
                          n716 = Less?(x=w1876, y=u8 100) -> (x < y?=w1878:bool)
                          n717 = case shown="False" w1878 {
                            tunnel: w1876 -> [w1890 w1977]
                            tunnel: [w1889 w1976] -> w1877
                            frame False {
                              n718 = Quotient & Remainder(x=w1890, y=u8 10) -> (x-y*floor(x/y)=w1888:u8, floor(x/y)=w1891:u8)
                              n719 = Subtract(x=w1891, y=u8 9) -> (x-y=w1893:u8)
                              n720 = Number To Decimal String(number=w1888) -> (decimal integer string=w1894:string)  [unwired: 1 in]
                              n721 = case shown="7" w1893 {
                                tunnel: w1894 -> [w1896 w1899 w1902 w1905 w1908 w1911 w1914 w1917 w1920 w1923 w1926 w1929 w1932 w1935 w1938 w1941 w1944 w1947 w1950 w1953 w1956 w1959 w1962 w1965 w1968 w1971 w1974]
                                tunnel: [w1895 w1898 w1901 w1904 w1907 w1910 w1913 w1916 w1919 w1922 w1925 w1928 w1931 w1934 w1937 w1940 w1943 w1946 w1949 w1952 w1955 w1958 w1961 w1964 w1967 w1970 w1973] -> w1889
                                frame 0, Default {
                                n722 = Concatenate Strings("0", w1896) -> (w1895:string)
                                }
                                frame 1 {
                                n723 = Concatenate Strings("A", w1899) -> (w1898:string)
                                }
                                frame 2 {
                                n724 = Concatenate Strings("B", w1902) -> (w1901:string)
                                }
                                frame 3 {
                                n725 = Concatenate Strings("C", w1905) -> (w1904:string)
                                }
                                frame 4 {
                                n726 = Concatenate Strings("D", w1908) -> (w1907:string)
                                }
                                frame 5 {
                                n727 = Concatenate Strings("E", w1911) -> (w1910:string)
                                }
                                frame 6 {
                                n728 = Concatenate Strings("F", w1914) -> (w1913:string)
                                }
                                frame 7 {
                                n729 = Concatenate Strings("G", w1917) -> (w1916:string)
                                }
                                frame 8 {
                                n730 = Concatenate Strings("H", w1920) -> (w1919:string)
                                }
                                frame 9 {
                                n731 = Concatenate Strings("I", w1923) -> (w1922:string)
                                }
                                frame 10 {
                                n732 = Concatenate Strings("J", w1926) -> (w1925:string)
                                }
                                frame 11 {
                                n733 = Concatenate Strings("K", w1929) -> (w1928:string)
                                }
                                frame 12 {
                                n734 = Concatenate Strings("L", w1932) -> (w1931:string)
                                }
                                frame 13 {
                                n735 = Concatenate Strings("M", w1935) -> (w1934:string)
                                }
                                frame 14 {
                                n736 = Concatenate Strings("N", w1938) -> (w1937:string)
                                }
                                frame 15 {
                                n737 = Concatenate Strings("O", w1941) -> (w1940:string)
                                }
                                frame 16 {
                                n738 = Concatenate Strings("P", w1944) -> (w1943:string)
                                }
                                frame 17 {
                                n739 = Concatenate Strings("Q", w1947) -> (w1946:string)
                                }
                                frame 18 {
                                n740 = Concatenate Strings("R", w1950) -> (w1949:string)
                                }
                                frame 19 {
                                n741 = Concatenate Strings("S", w1953) -> (w1952:string)
                                }
                                frame 20 {
                                n742 = Concatenate Strings("T", w1956) -> (w1955:string)
                                }
                                frame 21 {
                                n743 = Concatenate Strings("U", w1959) -> (w1958:string)
                                }
                                frame 22 {
                                n744 = Concatenate Strings("V", w1962) -> (w1961:string)
                                }
                                frame 23 {
                                n745 = Concatenate Strings("W", w1965) -> (w1964:string)
                                }
                                frame 24 {
                                n746 = Concatenate Strings("X", w1968) -> (w1967:string)
                                }
                                frame 25 {
                                n747 = Concatenate Strings("Y", w1971) -> (w1970:string)
                                }
                                frame 26 {
                                n748 = Concatenate Strings("Z", w1974) -> (w1973:string)
                                }
                              }
                            }
                            frame True {
                              n749 = Number To Decimal String(number=w1977) -> (decimal integer string=w1976:string)  [unwired: 1 in]
                            }
                          }
                          n750 = Concatenate Strings("$", w1881, w1877, "\r") -> (w1886:string)
                          n751 = VISA Write(VISA resource name=w1873, write buffer=w1886, error in (no error)=w1872) -> (VISA resource name out=w1875:refnum<visa-resource-name>, error out=w1874:errorcluster)  [unwired: 1 out]
                          n752 = VISA Close(VISA resource name=w1875, error in (no error)=w1874) -> ()  [unwired: 1 out]
                        }
                        frame #1 {
                          n753 = Wait Until Next ms Multiple(millisecond multiple=u32 300) -> ()  [unwired: 1 out]
                          n754 = Concatenate Strings(w1980, "63", w1978) -> (w1990:string)
                          n755 = String To Byte Array(string=w1990) -> (unsigned byte array=w1994:u8[])
                          n756 = Add Array Elements(numeric array=w1994) -> (sum=w1987:u8)
                          n757 = Less?(x=w1987, y=u8 100) -> (x < y?=w1989:bool)
                          n758 = case shown="False" w1989 {
                            tunnel: w1987 -> [w1998 w2085]
                            tunnel: [w1997 w2084] -> w1988
                            frame False {
                              n759 = Quotient & Remainder(x=w1998, y=u8 10) -> (x-y*floor(x/y)=w1996:u8, floor(x/y)=w1999:u8)
                              n760 = Subtract(x=w1999, y=u8 9) -> (x-y=w2001:u8)
                              n761 = Number To Decimal String(number=w1996) -> (decimal integer string=w2002:string)  [unwired: 1 in]
                              n762 = case shown="8" w2001 {
                                tunnel: w2002 -> [w2004 w2007 w2010 w2013 w2016 w2019 w2022 w2025 w2028 w2031 w2034 w2037 w2040 w2043 w2046 w2049 w2052 w2055 w2058 w2061 w2064 w2067 w2070 w2073 w2076 w2079 w2082]
                                tunnel: [w2003 w2006 w2009 w2012 w2015 w2018 w2021 w2024 w2027 w2030 w2033 w2036 w2039 w2042 w2045 w2048 w2051 w2054 w2057 w2060 w2063 w2066 w2069 w2072 w2075 w2078 w2081] -> w1997
                                frame 0, Default {
                                n763 = Concatenate Strings("0", w2004) -> (w2003:string)
                                }
                                frame 1 {
                                n764 = Concatenate Strings("A", w2007) -> (w2006:string)
                                }
                                frame 2 {
                                n765 = Concatenate Strings("B", w2010) -> (w2009:string)
                                }
                                frame 3 {
                                n766 = Concatenate Strings("C", w2013) -> (w2012:string)
                                }
                                frame 4 {
                                n767 = Concatenate Strings("D", w2016) -> (w2015:string)
                                }
                                frame 5 {
                                n768 = Concatenate Strings("E", w2019) -> (w2018:string)
                                }
                                frame 6 {
                                n769 = Concatenate Strings("F", w2022) -> (w2021:string)
                                }
                                frame 7 {
                                n770 = Concatenate Strings("G", w2025) -> (w2024:string)
                                }
                                frame 8 {
                                n771 = Concatenate Strings("H", w2028) -> (w2027:string)
                                }
                                frame 9 {
                                n772 = Concatenate Strings("I", w2031) -> (w2030:string)
                                }
                                frame 10 {
                                n773 = Concatenate Strings("J", w2034) -> (w2033:string)
                                }
                                frame 11 {
                                n774 = Concatenate Strings("K", w2037) -> (w2036:string)
                                }
                                frame 12 {
                                n775 = Concatenate Strings("L", w2040) -> (w2039:string)
                                }
                                frame 13 {
                                n776 = Concatenate Strings("M", w2043) -> (w2042:string)
                                }
                                frame 14 {
                                n777 = Concatenate Strings("N", w2046) -> (w2045:string)
                                }
                                frame 15 {
                                n778 = Concatenate Strings("O", w2049) -> (w2048:string)
                                }
                                frame 16 {
                                n779 = Concatenate Strings("P", w2052) -> (w2051:string)
                                }
                                frame 17 {
                                n780 = Concatenate Strings("Q", w2055) -> (w2054:string)
                                }
                                frame 18 {
                                n781 = Concatenate Strings("R", w2058) -> (w2057:string)
                                }
                                frame 19 {
                                n782 = Concatenate Strings("S", w2061) -> (w2060:string)
                                }
                                frame 20 {
                                n783 = Concatenate Strings("T", w2064) -> (w2063:string)
                                }
                                frame 21 {
                                n784 = Concatenate Strings("U", w2067) -> (w2066:string)
                                }
                                frame 22 {
                                n785 = Concatenate Strings("V", w2070) -> (w2069:string)
                                }
                                frame 23 {
                                n786 = Concatenate Strings("W", w2073) -> (w2072:string)
                                }
                                frame 24 {
                                n787 = Concatenate Strings("X", w2076) -> (w2075:string)
                                }
                                frame 25 {
                                n788 = Concatenate Strings("Y", w2079) -> (w2078:string)
                                }
                                frame 26 {
                                n789 = Concatenate Strings("Z", w2082) -> (w2081:string)
                                }
                              }
                            }
                            frame True {
                              n790 = Number To Decimal String(number=w2085) -> (decimal integer string=w2084:string)  [unwired: 1 in]
                            }
                          }
                          n791 = Concatenate Strings("$", w1990, w1988, "\r") -> (w1982:string)
                          n792 = VISA Write(VISA resource name=w1984, write buffer=w1982, error in (no error)=w1983) -> (VISA resource name out=w1986:refnum<visa-resource-name>, error out=w1985:errorcluster)  [unwired: 1 out]
                          n793 = VISA Close(VISA resource name=w1986, error in (no error)=w1985) -> ()  [unwired: 1 out]
                        }
                        frame #2 {
                          n794 = Wait Until Next ms Multiple(millisecond multiple=u32 300) -> ()  [unwired: 1 out]
                          n795 = Concatenate Strings("0101W71", w2087) -> (w2097:string)
                          n796 = String To Byte Array(string=w2097) -> (unsigned byte array=w2101:u8[])
                          n797 = Add Array Elements(numeric array=w2101) -> (sum=w2093:u8)
                          n798 = Less?(x=w2093, y=u8 100) -> (x < y?=w2095:bool)
                          n799 = case shown="False" w2095 {
                            tunnel: w2093 -> [w2105 w2192]
                            tunnel: [w2104 w2191] -> w2094
                            frame False {
                              n800 = Quotient & Remainder(x=w2105, y=u8 10) -> (x-y*floor(x/y)=w2103:u8, floor(x/y)=w2106:u8)
                              n801 = Subtract(x=w2106, y=u8 9) -> (x-y=w2108:u8)
                              n802 = Number To Decimal String(number=w2103) -> (decimal integer string=w2109:string)  [unwired: 1 in]
                              n803 = case shown="8" w2108 {
                                tunnel: w2109 -> [w2111 w2114 w2117 w2120 w2123 w2126 w2129 w2132 w2135 w2138 w2141 w2144 w2147 w2150 w2153 w2156 w2159 w2162 w2165 w2168 w2171 w2174 w2177 w2180 w2183 w2186 w2189]
                                tunnel: [w2110 w2113 w2116 w2119 w2122 w2125 w2128 w2131 w2134 w2137 w2140 w2143 w2146 w2149 w2152 w2155 w2158 w2161 w2164 w2167 w2170 w2173 w2176 w2179 w2182 w2185 w2188] -> w2104
                                frame 0, Default {
                                n804 = Concatenate Strings("0", w2111) -> (w2110:string)
                                }
                                frame 1 {
                                n805 = Concatenate Strings("A", w2114) -> (w2113:string)
                                }
                                frame 2 {
                                n806 = Concatenate Strings("B", w2117) -> (w2116:string)
                                }
                                frame 3 {
                                n807 = Concatenate Strings("C", w2120) -> (w2119:string)
                                }
                                frame 4 {
                                n808 = Concatenate Strings("D", w2123) -> (w2122:string)
                                }
                                frame 5 {
                                n809 = Concatenate Strings("E", w2126) -> (w2125:string)
                                }
                                frame 6 {
                                n810 = Concatenate Strings("F", w2129) -> (w2128:string)
                                }
                                frame 7 {
                                n811 = Concatenate Strings("G", w2132) -> (w2131:string)
                                }
                                frame 8 {
                                n812 = Concatenate Strings("H", w2135) -> (w2134:string)
                                }
                                frame 9 {
                                n813 = Concatenate Strings("I", w2138) -> (w2137:string)
                                }
                                frame 10 {
                                n814 = Concatenate Strings("J", w2141) -> (w2140:string)
                                }
                                frame 11 {
                                n815 = Concatenate Strings("K", w2144) -> (w2143:string)
                                }
                                frame 12 {
                                n816 = Concatenate Strings("L", w2147) -> (w2146:string)
                                }
                                frame 13 {
                                n817 = Concatenate Strings("M", w2150) -> (w2149:string)
                                }
                                frame 14 {
                                n818 = Concatenate Strings("N", w2153) -> (w2152:string)
                                }
                                frame 15 {
                                n819 = Concatenate Strings("O", w2156) -> (w2155:string)
                                }
                                frame 16 {
                                n820 = Concatenate Strings("P", w2159) -> (w2158:string)
                                }
                                frame 17 {
                                n821 = Concatenate Strings("Q", w2162) -> (w2161:string)
                                }
                                frame 18 {
                                n822 = Concatenate Strings("R", w2165) -> (w2164:string)
                                }
                                frame 19 {
                                n823 = Concatenate Strings("S", w2168) -> (w2167:string)
                                }
                                frame 20 {
                                n824 = Concatenate Strings("T", w2171) -> (w2170:string)
                                }
                                frame 21 {
                                n825 = Concatenate Strings("U", w2174) -> (w2173:string)
                                }
                                frame 22 {
                                n826 = Concatenate Strings("V", w2177) -> (w2176:string)
                                }
                                frame 23 {
                                n827 = Concatenate Strings("W", w2180) -> (w2179:string)
                                }
                                frame 24 {
                                n828 = Concatenate Strings("X", w2183) -> (w2182:string)
                                }
                                frame 25 {
                                n829 = Concatenate Strings("Y", w2186) -> (w2185:string)
                                }
                                frame 26 {
                                n830 = Concatenate Strings("Z", w2189) -> (w2188:string)
                                }
                              }
                            }
                            frame True {
                              n831 = Number To Decimal String(number=w2192) -> (decimal integer string=w2191:string)  [unwired: 1 in]
                            }
                          }
                          n832 = Concatenate Strings("$", w2097, w2094, "\r") -> (w2088:string)
                          n833 = VISA Write(VISA resource name=w2090, write buffer=w2088, error in (no error)=w2089) -> (VISA resource name out=w2092:refnum<visa-resource-name>, error out=w2091:errorcluster)  [unwired: 1 out]
                          n834 = VISA Close(VISA resource name=w2092, error in (no error)=w2091) -> ()  [unwired: 1 out]
                        }
                      }
                    }
                    frame 6 {
                      n835 = stacked-sequence {
                        tunnel: w2198 -> [w2207 _ _]
                        tunnel: w2197 -> [_ w2307 _]
                        tunnel: w2196 -> [w2201 w2312 w2418]
                        tunnel: w2195 -> [w2200 w2311 w2417]
                        tunnel: w2194 -> [_ _ w2415]
                        tunnel: w2193 -> [_ w2308 _]
                        frame #0 {
                          n836 = Wait Until Next ms Multiple(millisecond multiple=u32 300) -> ()  [unwired: 1 out]
                          n837 = Concatenate Strings("0101W48", w2207) -> (w2209:string)
                          n838 = String To Byte Array(string=w2209) -> (unsigned byte array=w2213:u8[])
                          n839 = Add Array Elements(numeric array=w2213) -> (sum=w2204:u8)
                          n840 = Less?(x=w2204, y=u8 100) -> (x < y?=w2206:bool)
                          n841 = case shown="False" w2206 {
                            tunnel: w2204 -> [w2218 w2305]
                            tunnel: [w2217 w2304] -> w2205
                            frame False {
                              n842 = Quotient & Remainder(x=w2218, y=u8 10) -> (x-y*floor(x/y)=w2216:u8, floor(x/y)=w2219:u8)
                              n843 = Subtract(x=w2219, y=u8 9) -> (x-y=w2221:u8)
                              n844 = Number To Decimal String(number=w2216) -> (decimal integer string=w2222:string)  [unwired: 1 in]
                              n845 = case shown="7" w2221 {
                                tunnel: w2222 -> [w2224 w2227 w2230 w2233 w2236 w2239 w2242 w2245 w2248 w2251 w2254 w2257 w2260 w2263 w2266 w2269 w2272 w2275 w2278 w2281 w2284 w2287 w2290 w2293 w2296 w2299 w2302]
                                tunnel: [w2223 w2226 w2229 w2232 w2235 w2238 w2241 w2244 w2247 w2250 w2253 w2256 w2259 w2262 w2265 w2268 w2271 w2274 w2277 w2280 w2283 w2286 w2289 w2292 w2295 w2298 w2301] -> w2217
                                frame 0, Default {
                                n846 = Concatenate Strings("0", w2224) -> (w2223:string)
                                }
                                frame 1 {
                                n847 = Concatenate Strings("A", w2227) -> (w2226:string)
                                }
                                frame 2 {
                                n848 = Concatenate Strings("B", w2230) -> (w2229:string)
                                }
                                frame 3 {
                                n849 = Concatenate Strings("C", w2233) -> (w2232:string)
                                }
                                frame 4 {
                                n850 = Concatenate Strings("D", w2236) -> (w2235:string)
                                }
                                frame 5 {
                                n851 = Concatenate Strings("E", w2239) -> (w2238:string)
                                }
                                frame 6 {
                                n852 = Concatenate Strings("F", w2242) -> (w2241:string)
                                }
                                frame 7 {
                                n853 = Concatenate Strings("G", w2245) -> (w2244:string)
                                }
                                frame 8 {
                                n854 = Concatenate Strings("H", w2248) -> (w2247:string)
                                }
                                frame 9 {
                                n855 = Concatenate Strings("I", w2251) -> (w2250:string)
                                }
                                frame 10 {
                                n856 = Concatenate Strings("J", w2254) -> (w2253:string)
                                }
                                frame 11 {
                                n857 = Concatenate Strings("K", w2257) -> (w2256:string)
                                }
                                frame 12 {
                                n858 = Concatenate Strings("L", w2260) -> (w2259:string)
                                }
                                frame 13 {
                                n859 = Concatenate Strings("M", w2263) -> (w2262:string)
                                }
                                frame 14 {
                                n860 = Concatenate Strings("N", w2266) -> (w2265:string)
                                }
                                frame 15 {
                                n861 = Concatenate Strings("O", w2269) -> (w2268:string)
                                }
                                frame 16 {
                                n862 = Concatenate Strings("P", w2272) -> (w2271:string)
                                }
                                frame 17 {
                                n863 = Concatenate Strings("Q", w2275) -> (w2274:string)
                                }
                                frame 18 {
                                n864 = Concatenate Strings("R", w2278) -> (w2277:string)
                                }
                                frame 19 {
                                n865 = Concatenate Strings("S", w2281) -> (w2280:string)
                                }
                                frame 20 {
                                n866 = Concatenate Strings("T", w2284) -> (w2283:string)
                                }
                                frame 21 {
                                n867 = Concatenate Strings("U", w2287) -> (w2286:string)
                                }
                                frame 22 {
                                n868 = Concatenate Strings("V", w2290) -> (w2289:string)
                                }
                                frame 23 {
                                n869 = Concatenate Strings("W", w2293) -> (w2292:string)
                                }
                                frame 24 {
                                n870 = Concatenate Strings("X", w2296) -> (w2295:string)
                                }
                                frame 25 {
                                n871 = Concatenate Strings("Y", w2299) -> (w2298:string)
                                }
                                frame 26 {
                                n872 = Concatenate Strings("Z", w2302) -> (w2301:string)
                                }
                              }
                            }
                            frame True {
                              n873 = Number To Decimal String(number=w2305) -> (decimal integer string=w2304:string)  [unwired: 1 in]
                            }
                          }
                          n874 = Concatenate Strings("$", w2209, w2205, "\r") -> (w2214:string)
                          n875 = VISA Write(VISA resource name=w2201, write buffer=w2214, error in (no error)=w2200) -> (VISA resource name out=w2203:refnum<visa-resource-name>, error out=w2202:errorcluster)  [unwired: 1 out]
                          n876 = VISA Close(VISA resource name=w2203, error in (no error)=w2202) -> ()  [unwired: 1 out]
                        }
                        frame #1 {
                          n877 = Wait Until Next ms Multiple(millisecond multiple=u32 300) -> ()  [unwired: 1 out]
                          n878 = Concatenate Strings(w2308, "64", w2307) -> (w2318:string)
                          n879 = String To Byte Array(string=w2318) -> (unsigned byte array=w2322:u8[])
                          n880 = Add Array Elements(numeric array=w2322) -> (sum=w2315:u8)
                          n881 = Less?(x=w2315, y=u8 100) -> (x < y?=w2317:bool)
                          n882 = case shown="False" w2317 {
                            tunnel: w2315 -> [w2326 w2413]
                            tunnel: [w2325 w2412] -> w2316
                            frame False {
                              n883 = Quotient & Remainder(x=w2326, y=u8 10) -> (x-y*floor(x/y)=w2324:u8, floor(x/y)=w2327:u8)
                              n884 = Subtract(x=w2327, y=u8 9) -> (x-y=w2329:u8)
                              n885 = Number To Decimal String(number=w2324) -> (decimal integer string=w2330:string)  [unwired: 1 in]
                              n886 = case shown="8" w2329 {
                                tunnel: w2330 -> [w2332 w2335 w2338 w2341 w2344 w2347 w2350 w2353 w2356 w2359 w2362 w2365 w2368 w2371 w2374 w2377 w2380 w2383 w2386 w2389 w2392 w2395 w2398 w2401 w2404 w2407 w2410]
                                tunnel: [w2331 w2334 w2337 w2340 w2343 w2346 w2349 w2352 w2355 w2358 w2361 w2364 w2367 w2370 w2373 w2376 w2379 w2382 w2385 w2388 w2391 w2394 w2397 w2400 w2403 w2406 w2409] -> w2325
                                frame 0, Default {
                                n887 = Concatenate Strings("0", w2332) -> (w2331:string)
                                }
                                frame 1 {
                                n888 = Concatenate Strings("A", w2335) -> (w2334:string)
                                }
                                frame 2 {
                                n889 = Concatenate Strings("B", w2338) -> (w2337:string)
                                }
                                frame 3 {
                                n890 = Concatenate Strings("C", w2341) -> (w2340:string)
                                }
                                frame 4 {
                                n891 = Concatenate Strings("D", w2344) -> (w2343:string)
                                }
                                frame 5 {
                                n892 = Concatenate Strings("E", w2347) -> (w2346:string)
                                }
                                frame 6 {
                                n893 = Concatenate Strings("F", w2350) -> (w2349:string)
                                }
                                frame 7 {
                                n894 = Concatenate Strings("G", w2353) -> (w2352:string)
                                }
                                frame 8 {
                                n895 = Concatenate Strings("H", w2356) -> (w2355:string)
                                }
                                frame 9 {
                                n896 = Concatenate Strings("I", w2359) -> (w2358:string)
                                }
                                frame 10 {
                                n897 = Concatenate Strings("J", w2362) -> (w2361:string)
                                }
                                frame 11 {
                                n898 = Concatenate Strings("K", w2365) -> (w2364:string)
                                }
                                frame 12 {
                                n899 = Concatenate Strings("L", w2368) -> (w2367:string)
                                }
                                frame 13 {
                                n900 = Concatenate Strings("M", w2371) -> (w2370:string)
                                }
                                frame 14 {
                                n901 = Concatenate Strings("N", w2374) -> (w2373:string)
                                }
                                frame 15 {
                                n902 = Concatenate Strings("O", w2377) -> (w2376:string)
                                }
                                frame 16 {
                                n903 = Concatenate Strings("P", w2380) -> (w2379:string)
                                }
                                frame 17 {
                                n904 = Concatenate Strings("Q", w2383) -> (w2382:string)
                                }
                                frame 18 {
                                n905 = Concatenate Strings("R", w2386) -> (w2385:string)
                                }
                                frame 19 {
                                n906 = Concatenate Strings("S", w2389) -> (w2388:string)
                                }
                                frame 20 {
                                n907 = Concatenate Strings("T", w2392) -> (w2391:string)
                                }
                                frame 21 {
                                n908 = Concatenate Strings("U", w2395) -> (w2394:string)
                                }
                                frame 22 {
                                n909 = Concatenate Strings("V", w2398) -> (w2397:string)
                                }
                                frame 23 {
                                n910 = Concatenate Strings("W", w2401) -> (w2400:string)
                                }
                                frame 24 {
                                n911 = Concatenate Strings("X", w2404) -> (w2403:string)
                                }
                                frame 25 {
                                n912 = Concatenate Strings("Y", w2407) -> (w2406:string)
                                }
                                frame 26 {
                                n913 = Concatenate Strings("Z", w2410) -> (w2409:string)
                                }
                              }
                            }
                            frame True {
                              n914 = Number To Decimal String(number=w2413) -> (decimal integer string=w2412:string)  [unwired: 1 in]
                            }
                          }
                          n915 = Concatenate Strings("$", w2318, w2316, "\r") -> (w2310:string)
                          n916 = VISA Write(VISA resource name=w2312, write buffer=w2310, error in (no error)=w2311) -> (VISA resource name out=w2314:refnum<visa-resource-name>, error out=w2313:errorcluster)  [unwired: 1 out]
                          n917 = VISA Close(VISA resource name=w2314, error in (no error)=w2313) -> ()  [unwired: 1 out]
                        }
                        frame #2 {
                          n918 = Wait Until Next ms Multiple(millisecond multiple=u32 300) -> ()  [unwired: 1 out]
                          n919 = Concatenate Strings("0101W72", w2415) -> (w2425:string)
                          n920 = String To Byte Array(string=w2425) -> (unsigned byte array=w2429:u8[])
                          n921 = Add Array Elements(numeric array=w2429) -> (sum=w2421:u8)
                          n922 = Less?(x=w2421, y=u8 100) -> (x < y?=w2423:bool)
                          n923 = case shown="False" w2423 {
                            tunnel: w2421 -> [w2433 w2520]
                            tunnel: [w2432 w2519] -> w2422
                            frame False {
                              n924 = Quotient & Remainder(x=w2433, y=u8 10) -> (x-y*floor(x/y)=w2431:u8, floor(x/y)=w2434:u8)
                              n925 = Subtract(x=w2434, y=u8 9) -> (x-y=w2436:u8)
                              n926 = Number To Decimal String(number=w2431) -> (decimal integer string=w2437:string)  [unwired: 1 in]
                              n927 = case shown="8" w2436 {
                                tunnel: w2437 -> [w2439 w2442 w2445 w2448 w2451 w2454 w2457 w2460 w2463 w2466 w2469 w2472 w2475 w2478 w2481 w2484 w2487 w2490 w2493 w2496 w2499 w2502 w2505 w2508 w2511 w2514 w2517]
                                tunnel: [w2438 w2441 w2444 w2447 w2450 w2453 w2456 w2459 w2462 w2465 w2468 w2471 w2474 w2477 w2480 w2483 w2486 w2489 w2492 w2495 w2498 w2501 w2504 w2507 w2510 w2513 w2516] -> w2432
                                frame 0, Default {
                                n928 = Concatenate Strings("0", w2439) -> (w2438:string)
                                }
                                frame 1 {
                                n929 = Concatenate Strings("A", w2442) -> (w2441:string)
                                }
                                frame 2 {
                                n930 = Concatenate Strings("B", w2445) -> (w2444:string)
                                }
                                frame 3 {
                                n931 = Concatenate Strings("C", w2448) -> (w2447:string)
                                }
                                frame 4 {
                                n932 = Concatenate Strings("D", w2451) -> (w2450:string)
                                }
                                frame 5 {
                                n933 = Concatenate Strings("E", w2454) -> (w2453:string)
                                }
                                frame 6 {
                                n934 = Concatenate Strings("F", w2457) -> (w2456:string)
                                }
                                frame 7 {
                                n935 = Concatenate Strings("G", w2460) -> (w2459:string)
                                }
                                frame 8 {
                                n936 = Concatenate Strings("H", w2463) -> (w2462:string)
                                }
                                frame 9 {
                                n937 = Concatenate Strings("I", w2466) -> (w2465:string)
                                }
                                frame 10 {
                                n938 = Concatenate Strings("J", w2469) -> (w2468:string)
                                }
                                frame 11 {
                                n939 = Concatenate Strings("K", w2472) -> (w2471:string)
                                }
                                frame 12 {
                                n940 = Concatenate Strings("L", w2475) -> (w2474:string)
                                }
                                frame 13 {
                                n941 = Concatenate Strings("M", w2478) -> (w2477:string)
                                }
                                frame 14 {
                                n942 = Concatenate Strings("N", w2481) -> (w2480:string)
                                }
                                frame 15 {
                                n943 = Concatenate Strings("O", w2484) -> (w2483:string)
                                }
                                frame 16 {
                                n944 = Concatenate Strings("P", w2487) -> (w2486:string)
                                }
                                frame 17 {
                                n945 = Concatenate Strings("Q", w2490) -> (w2489:string)
                                }
                                frame 18 {
                                n946 = Concatenate Strings("R", w2493) -> (w2492:string)
                                }
                                frame 19 {
                                n947 = Concatenate Strings("S", w2496) -> (w2495:string)
                                }
                                frame 20 {
                                n948 = Concatenate Strings("T", w2499) -> (w2498:string)
                                }
                                frame 21 {
                                n949 = Concatenate Strings("U", w2502) -> (w2501:string)
                                }
                                frame 22 {
                                n950 = Concatenate Strings("V", w2505) -> (w2504:string)
                                }
                                frame 23 {
                                n951 = Concatenate Strings("W", w2508) -> (w2507:string)
                                }
                                frame 24 {
                                n952 = Concatenate Strings("X", w2511) -> (w2510:string)
                                }
                                frame 25 {
                                n953 = Concatenate Strings("Y", w2514) -> (w2513:string)
                                }
                                frame 26 {
                                n954 = Concatenate Strings("Z", w2517) -> (w2516:string)
                                }
                              }
                            }
                            frame True {
                              n955 = Number To Decimal String(number=w2520) -> (decimal integer string=w2519:string)  [unwired: 1 in]
                            }
                          }
                          n956 = Concatenate Strings("$", w2425, w2422, "\r") -> (w2416:string)
                          n957 = VISA Write(VISA resource name=w2418, write buffer=w2416, error in (no error)=w2417) -> (VISA resource name out=w2420:refnum<visa-resource-name>, error out=w2419:errorcluster)  [unwired: 1 out]
                          n958 = VISA Close(VISA resource name=w2420, error in (no error)=w2419) -> ()  [unwired: 1 out]
                        }
                      }
                    }
                    frame 7 {
                      n959 = stacked-sequence {
                        tunnel: w2526 -> [w2535 _ _]
                        tunnel: w2525 -> [_ w2636 _]
                        tunnel: w2524 -> [w2529 w2640 w2746]
                        tunnel: w2523 -> [w2528 w2639 w2745]
                        tunnel: w2522 -> [_ _ w2743]
                        tunnel: w2521 -> [_ w2634 _]
                        frame #0 {
                          n960 = Wait Until Next ms Multiple(millisecond multiple=u32 300) -> ()  [unwired: 1 out]
                          n961 = Concatenate Strings("0101W49", w2535) -> (w2537:string)
                          n962 = String To Byte Array(string=w2537) -> (unsigned byte array=w2541:u8[])
                          n963 = Add Array Elements(numeric array=w2541) -> (sum=w2532:u8)
                          n964 = Less?(x=w2532, y=u8 100) -> (x < y?=w2534:bool)
                          n965 = case shown="False" w2534 {
                            tunnel: w2532 -> [w2546 w2633]
                            tunnel: [w2545 w2632] -> w2533
                            frame False {
                              n966 = Quotient & Remainder(x=w2546, y=u8 10) -> (x-y*floor(x/y)=w2544:u8, floor(x/y)=w2547:u8)
                              n967 = Subtract(x=w2547, y=u8 9) -> (x-y=w2549:u8)
                              n968 = Number To Decimal String(number=w2544) -> (decimal integer string=w2550:string)  [unwired: 1 in]
                              n969 = case shown="7" w2549 {
                                tunnel: w2550 -> [w2552 w2555 w2558 w2561 w2564 w2567 w2570 w2573 w2576 w2579 w2582 w2585 w2588 w2591 w2594 w2597 w2600 w2603 w2606 w2609 w2612 w2615 w2618 w2621 w2624 w2627 w2630]
                                tunnel: [w2551 w2554 w2557 w2560 w2563 w2566 w2569 w2572 w2575 w2578 w2581 w2584 w2587 w2590 w2593 w2596 w2599 w2602 w2605 w2608 w2611 w2614 w2617 w2620 w2623 w2626 w2629] -> w2545
                                frame 0, Default {
                                n970 = Concatenate Strings("0", w2552) -> (w2551:string)
                                }
                                frame 1 {
                                n971 = Concatenate Strings("A", w2555) -> (w2554:string)
                                }
                                frame 2 {
                                n972 = Concatenate Strings("B", w2558) -> (w2557:string)
                                }
                                frame 3 {
                                n973 = Concatenate Strings("C", w2561) -> (w2560:string)
                                }
                                frame 4 {
                                n974 = Concatenate Strings("D", w2564) -> (w2563:string)
                                }
                                frame 5 {
                                n975 = Concatenate Strings("E", w2567) -> (w2566:string)
                                }
                                frame 6 {
                                n976 = Concatenate Strings("F", w2570) -> (w2569:string)
                                }
                                frame 7 {
                                n977 = Concatenate Strings("G", w2573) -> (w2572:string)
                                }
                                frame 8 {
                                n978 = Concatenate Strings("H", w2576) -> (w2575:string)
                                }
                                frame 9 {
                                n979 = Concatenate Strings("I", w2579) -> (w2578:string)
                                }
                                frame 10 {
                                n980 = Concatenate Strings("J", w2582) -> (w2581:string)
                                }
                                frame 11 {
                                n981 = Concatenate Strings("K", w2585) -> (w2584:string)
                                }
                                frame 12 {
                                n982 = Concatenate Strings("L", w2588) -> (w2587:string)
                                }
                                frame 13 {
                                n983 = Concatenate Strings("M", w2591) -> (w2590:string)
                                }
                                frame 14 {
                                n984 = Concatenate Strings("N", w2594) -> (w2593:string)
                                }
                                frame 15 {
                                n985 = Concatenate Strings("O", w2597) -> (w2596:string)
                                }
                                frame 16 {
                                n986 = Concatenate Strings("P", w2600) -> (w2599:string)
                                }
                                frame 17 {
                                n987 = Concatenate Strings("Q", w2603) -> (w2602:string)
                                }
                                frame 18 {
                                n988 = Concatenate Strings("R", w2606) -> (w2605:string)
                                }
                                frame 19 {
                                n989 = Concatenate Strings("S", w2609) -> (w2608:string)
                                }
                                frame 20 {
                                n990 = Concatenate Strings("T", w2612) -> (w2611:string)
                                }
                                frame 21 {
                                n991 = Concatenate Strings("U", w2615) -> (w2614:string)
                                }
                                frame 22 {
                                n992 = Concatenate Strings("V", w2618) -> (w2617:string)
                                }
                                frame 23 {
                                n993 = Concatenate Strings("W", w2621) -> (w2620:string)
                                }
                                frame 24 {
                                n994 = Concatenate Strings("X", w2624) -> (w2623:string)
                                }
                                frame 25 {
                                n995 = Concatenate Strings("Y", w2627) -> (w2626:string)
                                }
                                frame 26 {
                                n996 = Concatenate Strings("Z", w2630) -> (w2629:string)
                                }
                              }
                            }
                            frame True {
                              n997 = Number To Decimal String(number=w2633) -> (decimal integer string=w2632:string)  [unwired: 1 in]
                            }
                          }
                          n998 = Concatenate Strings("$", w2537, w2533, "\r") -> (w2542:string)
                          n999 = VISA Write(VISA resource name=w2529, write buffer=w2542, error in (no error)=w2528) -> (VISA resource name out=w2531:refnum<visa-resource-name>, error out=w2530:errorcluster)  [unwired: 1 out]
                          n1000 = VISA Close(VISA resource name=w2531, error in (no error)=w2530) -> ()  [unwired: 1 out]
                        }
                        frame #1 {
                          n1001 = Wait Until Next ms Multiple(millisecond multiple=u32 300) -> ()  [unwired: 1 out]
                          n1002 = Concatenate Strings(w2634, "65", w2636) -> (w2646:string)
                          n1003 = String To Byte Array(string=w2646) -> (unsigned byte array=w2650:u8[])
                          n1004 = Add Array Elements(numeric array=w2650) -> (sum=w2643:u8)
                          n1005 = Less?(x=w2643, y=u8 100) -> (x < y?=w2645:bool)
                          n1006 = case shown="False" w2645 {
                            tunnel: w2643 -> [w2654 w2741]
                            tunnel: [w2653 w2740] -> w2644
                            frame False {
                              n1007 = Quotient & Remainder(x=w2654, y=u8 10) -> (x-y*floor(x/y)=w2652:u8, floor(x/y)=w2655:u8)
                              n1008 = Subtract(x=w2655, y=u8 9) -> (x-y=w2657:u8)
                              n1009 = Number To Decimal String(number=w2652) -> (decimal integer string=w2658:string)  [unwired: 1 in]
                              n1010 = case shown="8" w2657 {
                                tunnel: w2658 -> [w2660 w2663 w2666 w2669 w2672 w2675 w2678 w2681 w2684 w2687 w2690 w2693 w2696 w2699 w2702 w2705 w2708 w2711 w2714 w2717 w2720 w2723 w2726 w2729 w2732 w2735 w2738]
                                tunnel: [w2659 w2662 w2665 w2668 w2671 w2674 w2677 w2680 w2683 w2686 w2689 w2692 w2695 w2698 w2701 w2704 w2707 w2710 w2713 w2716 w2719 w2722 w2725 w2728 w2731 w2734 w2737] -> w2653
                                frame 0, Default {
                                n1011 = Concatenate Strings("0", w2660) -> (w2659:string)
                                }
                                frame 1 {
                                n1012 = Concatenate Strings("A", w2663) -> (w2662:string)
                                }
                                frame 2 {
                                n1013 = Concatenate Strings("B", w2666) -> (w2665:string)
                                }
                                frame 3 {
                                n1014 = Concatenate Strings("C", w2669) -> (w2668:string)
                                }
                                frame 4 {
                                n1015 = Concatenate Strings("D", w2672) -> (w2671:string)
                                }
                                frame 5 {
                                n1016 = Concatenate Strings("E", w2675) -> (w2674:string)
                                }
                                frame 6 {
                                n1017 = Concatenate Strings("F", w2678) -> (w2677:string)
                                }
                                frame 7 {
                                n1018 = Concatenate Strings("G", w2681) -> (w2680:string)
                                }
                                frame 8 {
                                n1019 = Concatenate Strings("H", w2684) -> (w2683:string)
                                }
                                frame 9 {
                                n1020 = Concatenate Strings("I", w2687) -> (w2686:string)
                                }
                                frame 10 {
                                n1021 = Concatenate Strings("J", w2690) -> (w2689:string)
                                }
                                frame 11 {
                                n1022 = Concatenate Strings("K", w2693) -> (w2692:string)
                                }
                                frame 12 {
                                n1023 = Concatenate Strings("L", w2696) -> (w2695:string)
                                }
                                frame 13 {
                                n1024 = Concatenate Strings("M", w2699) -> (w2698:string)
                                }
                                frame 14 {
                                n1025 = Concatenate Strings("N", w2702) -> (w2701:string)
                                }
                                frame 15 {
                                n1026 = Concatenate Strings("O", w2705) -> (w2704:string)
                                }
                                frame 16 {
                                n1027 = Concatenate Strings("P", w2708) -> (w2707:string)
                                }
                                frame 17 {
                                n1028 = Concatenate Strings("Q", w2711) -> (w2710:string)
                                }
                                frame 18 {
                                n1029 = Concatenate Strings("R", w2714) -> (w2713:string)
                                }
                                frame 19 {
                                n1030 = Concatenate Strings("S", w2717) -> (w2716:string)
                                }
                                frame 20 {
                                n1031 = Concatenate Strings("T", w2720) -> (w2719:string)
                                }
                                frame 21 {
                                n1032 = Concatenate Strings("U", w2723) -> (w2722:string)
                                }
                                frame 22 {
                                n1033 = Concatenate Strings("V", w2726) -> (w2725:string)
                                }
                                frame 23 {
                                n1034 = Concatenate Strings("W", w2729) -> (w2728:string)
                                }
                                frame 24 {
                                n1035 = Concatenate Strings("X", w2732) -> (w2731:string)
                                }
                                frame 25 {
                                n1036 = Concatenate Strings("Y", w2735) -> (w2734:string)
                                }
                                frame 26 {
                                n1037 = Concatenate Strings("Z", w2738) -> (w2737:string)
                                }
                              }
                            }
                            frame True {
                              n1038 = Number To Decimal String(number=w2741) -> (decimal integer string=w2740:string)  [unwired: 1 in]
                            }
                          }
                          n1039 = Concatenate Strings("$", w2646, w2644, "\r") -> (w2638:string)
                          n1040 = VISA Write(VISA resource name=w2640, write buffer=w2638, error in (no error)=w2639) -> (VISA resource name out=w2642:refnum<visa-resource-name>, error out=w2641:errorcluster)  [unwired: 1 out]
                          n1041 = VISA Close(VISA resource name=w2642, error in (no error)=w2641) -> ()  [unwired: 1 out]
                        }
                        frame #2 {
                          n1042 = Wait Until Next ms Multiple(millisecond multiple=u32 300) -> ()  [unwired: 1 out]
                          n1043 = Concatenate Strings("0101W73", w2743) -> (w2753:string)
                          n1044 = String To Byte Array(string=w2753) -> (unsigned byte array=w2757:u8[])
                          n1045 = Add Array Elements(numeric array=w2757) -> (sum=w2749:u8)
                          n1046 = Less?(x=w2749, y=u8 100) -> (x < y?=w2751:bool)
                          n1047 = case shown="False" w2751 {
                            tunnel: w2749 -> [w2761 w2848]
                            tunnel: [w2760 w2847] -> w2750
                            frame False {
                              n1048 = Quotient & Remainder(x=w2761, y=u8 10) -> (x-y*floor(x/y)=w2759:u8, floor(x/y)=w2762:u8)
                              n1049 = Subtract(x=w2762, y=u8 9) -> (x-y=w2764:u8)
                              n1050 = Number To Decimal String(number=w2759) -> (decimal integer string=w2765:string)  [unwired: 1 in]
                              n1051 = case shown="8" w2764 {
                                tunnel: w2765 -> [w2767 w2770 w2773 w2776 w2779 w2782 w2785 w2788 w2791 w2794 w2797 w2800 w2803 w2806 w2809 w2812 w2815 w2818 w2821 w2824 w2827 w2830 w2833 w2836 w2839 w2842 w2845]
                                tunnel: [w2766 w2769 w2772 w2775 w2778 w2781 w2784 w2787 w2790 w2793 w2796 w2799 w2802 w2805 w2808 w2811 w2814 w2817 w2820 w2823 w2826 w2829 w2832 w2835 w2838 w2841 w2844] -> w2760
                                frame 0, Default {
                                n1052 = Concatenate Strings("0", w2767) -> (w2766:string)
                                }
                                frame 1 {
                                n1053 = Concatenate Strings("A", w2770) -> (w2769:string)
                                }
                                frame 2 {
                                n1054 = Concatenate Strings("B", w2773) -> (w2772:string)
                                }
                                frame 3 {
                                n1055 = Concatenate Strings("C", w2776) -> (w2775:string)
                                }
                                frame 4 {
                                n1056 = Concatenate Strings("D", w2779) -> (w2778:string)
                                }
                                frame 5 {
                                n1057 = Concatenate Strings("E", w2782) -> (w2781:string)
                                }
                                frame 6 {
                                n1058 = Concatenate Strings("F", w2785) -> (w2784:string)
                                }
                                frame 7 {
                                n1059 = Concatenate Strings("G", w2788) -> (w2787:string)
                                }
                                frame 8 {
                                n1060 = Concatenate Strings("H", w2791) -> (w2790:string)
                                }
                                frame 9 {
                                n1061 = Concatenate Strings("I", w2794) -> (w2793:string)
                                }
                                frame 10 {
                                n1062 = Concatenate Strings("J", w2797) -> (w2796:string)
                                }
                                frame 11 {
                                n1063 = Concatenate Strings("K", w2800) -> (w2799:string)
                                }
                                frame 12 {
                                n1064 = Concatenate Strings("L", w2803) -> (w2802:string)
                                }
                                frame 13 {
                                n1065 = Concatenate Strings("M", w2806) -> (w2805:string)
                                }
                                frame 14 {
                                n1066 = Concatenate Strings("N", w2809) -> (w2808:string)
                                }
                                frame 15 {
                                n1067 = Concatenate Strings("O", w2812) -> (w2811:string)
                                }
                                frame 16 {
                                n1068 = Concatenate Strings("P", w2815) -> (w2814:string)
                                }
                                frame 17 {
                                n1069 = Concatenate Strings("Q", w2818) -> (w2817:string)
                                }
                                frame 18 {
                                n1070 = Concatenate Strings("R", w2821) -> (w2820:string)
                                }
                                frame 19 {
                                n1071 = Concatenate Strings("S", w2824) -> (w2823:string)
                                }
                                frame 20 {
                                n1072 = Concatenate Strings("T", w2827) -> (w2826:string)
                                }
                                frame 21 {
                                n1073 = Concatenate Strings("U", w2830) -> (w2829:string)
                                }
                                frame 22 {
                                n1074 = Concatenate Strings("V", w2833) -> (w2832:string)
                                }
                                frame 23 {
                                n1075 = Concatenate Strings("W", w2836) -> (w2835:string)
                                }
                                frame 24 {
                                n1076 = Concatenate Strings("X", w2839) -> (w2838:string)
                                }
                                frame 25 {
                                n1077 = Concatenate Strings("Y", w2842) -> (w2841:string)
                                }
                                frame 26 {
                                n1078 = Concatenate Strings("Z", w2845) -> (w2844:string)
                                }
                              }
                            }
                            frame True {
                              n1079 = Number To Decimal String(number=w2848) -> (decimal integer string=w2847:string)  [unwired: 1 in]
                            }
                          }
                          n1080 = Concatenate Strings("$", w2753, w2750, "\r") -> (w2744:string)
                          n1081 = VISA Write(VISA resource name=w2746, write buffer=w2744, error in (no error)=w2745) -> (VISA resource name out=w2748:refnum<visa-resource-name>, error out=w2747:errorcluster)  [unwired: 1 out]
                          n1082 = VISA Close(VISA resource name=w2748, error in (no error)=w2747) -> ()  [unwired: 1 out]
                        }
                      }
                    }
                  }
                }
              }
              frame #1 {
                n1083 = stacked-sequence {
                  tunnel: w2850 -> [w2853 w2965]
                  tunnel: w2849 -> [w2852 w2964]
                  frame #0 {
                    n1084 = Number To Fractional String(number="Holdback (deg C)", width (-)=i16 5) -> (F-format string=w2862:string)  [unwired: 2 in]
                    n1085 = String Subset(string=w2862, length (rest)=6 ("length (rest)")) -> (substring=w2857:string)  [unwired: 1 in]
                    n1086 = Concatenate Strings("0101W83", w2857) -> (w2856:string)
                    n1087 = String To Byte Array(string=w2856) -> (unsigned byte array=w2869:u8[])
                    n1088 = Add Array Elements(numeric array=w2869) -> (sum=w2860:u8)
                    n1089 = Less?(x=w2860, y=u8 100) -> (x < y?=w2867:bool)
                    n1090 = case shown="False" w2867 {
                      tunnel: w2860 -> [w2874 w2961]
                      tunnel: [w2873 w2960] -> w2865
                      frame False {
                        n1091 = Quotient & Remainder(x=w2874, y=u8 10) -> (x-y*floor(x/y)=w2872:u8, floor(x/y)=w2875:u8)
                        n1092 = Subtract(x=w2875, y=u8 9) -> (x-y=w2877:u8)
                        n1093 = Number To Decimal String(number=w2872) -> (decimal integer string=w2878:string)  [unwired: 1 in]
                        n1094 = case shown="8" w2877 {
                          tunnel: w2878 -> [w2880 w2883 w2886 w2889 w2892 w2895 w2898 w2901 w2904 w2907 w2910 w2913 w2916 w2919 w2922 w2925 w2928 w2931 w2934 w2937 w2940 w2943 w2946 w2949 w2952 w2955 w2958]
                          tunnel: [w2879 w2882 w2885 w2888 w2891 w2894 w2897 w2900 w2903 w2906 w2909 w2912 w2915 w2918 w2921 w2924 w2927 w2930 w2933 w2936 w2939 w2942 w2945 w2948 w2951 w2954 w2957] -> w2873
                          frame 0, Default {
                            n1095 = Concatenate Strings("0", w2880) -> (w2879:string)
                          }
                          frame 1 {
                            n1096 = Concatenate Strings("A", w2883) -> (w2882:string)
                          }
                          frame 2 {
                            n1097 = Concatenate Strings("B", w2886) -> (w2885:string)
                          }
                          frame 3 {
                            n1098 = Concatenate Strings("C", w2889) -> (w2888:string)
                          }
                          frame 4 {
                            n1099 = Concatenate Strings("D", w2892) -> (w2891:string)
                          }
                          frame 5 {
                            n1100 = Concatenate Strings("E", w2895) -> (w2894:string)
                          }
                          frame 6 {
                            n1101 = Concatenate Strings("F", w2898) -> (w2897:string)
                          }
                          frame 7 {
                            n1102 = Concatenate Strings("G", w2901) -> (w2900:string)
                          }
                          frame 8 {
                            n1103 = Concatenate Strings("H", w2904) -> (w2903:string)
                          }
                          frame 9 {
                            n1104 = Concatenate Strings("I", w2907) -> (w2906:string)
                          }
                          frame 10 {
                            n1105 = Concatenate Strings("J", w2910) -> (w2909:string)
                          }
                          frame 11 {
                            n1106 = Concatenate Strings("K", w2913) -> (w2912:string)
                          }
                          frame 12 {
                            n1107 = Concatenate Strings("L", w2916) -> (w2915:string)
                          }
                          frame 13 {
                            n1108 = Concatenate Strings("M", w2919) -> (w2918:string)
                          }
                          frame 14 {
                            n1109 = Concatenate Strings("N", w2922) -> (w2921:string)
                          }
                          frame 15 {
                            n1110 = Concatenate Strings("O", w2925) -> (w2924:string)
                          }
                          frame 16 {
                            n1111 = Concatenate Strings("P", w2928) -> (w2927:string)
                          }
                          frame 17 {
                            n1112 = Concatenate Strings("Q", w2931) -> (w2930:string)
                          }
                          frame 18 {
                            n1113 = Concatenate Strings("R", w2934) -> (w2933:string)
                          }
                          frame 19 {
                            n1114 = Concatenate Strings("S", w2937) -> (w2936:string)
                          }
                          frame 20 {
                            n1115 = Concatenate Strings("T", w2940) -> (w2939:string)
                          }
                          frame 21 {
                            n1116 = Concatenate Strings("U", w2943) -> (w2942:string)
                          }
                          frame 22 {
                            n1117 = Concatenate Strings("V", w2946) -> (w2945:string)
                          }
                          frame 23 {
                            n1118 = Concatenate Strings("W", w2949) -> (w2948:string)
                          }
                          frame 24 {
                            n1119 = Concatenate Strings("X", w2952) -> (w2951:string)
                          }
                          frame 25 {
                            n1120 = Concatenate Strings("Y", w2955) -> (w2954:string)
                          }
                          frame 26 {
                            n1121 = Concatenate Strings("Z", w2958) -> (w2957:string)
                          }
                        }
                      }
                      frame True {
                        n1122 = Number To Decimal String(number=w2961) -> (decimal integer string=w2960:string)  [unwired: 1 in]
                      }
                    }
                    n1123 = Concatenate Strings("$", w2856, w2865, "\r") -> (w2870:string)
                    n1124 = VISA Write(VISA resource name=w2853, write buffer=w2870, error in (no error)=w2852) -> (VISA resource name out=w2859:refnum<visa-resource-name>, error out=w2858:errorcluster)  [unwired: 1 out]
                    n1125 = Wait Until Next ms Multiple(millisecond multiple=u32 300) -> ()  [unwired: 1 out]
                    n1126 = VISA Close(VISA resource name=w2859, error in (no error)=w2858) -> ()  [unwired: 1 out]
                  }
                  frame #1 {
                    n1127 = Number To Fractional String(number="Recycle #", width (-)=i16 5) -> (F-format string=w2973:string)  [unwired: 2 in]
                    n1128 = String Subset(string=w2973, length (rest)=6 ("length (rest)")) -> (substring=w2968:string)  [unwired: 1 in]
                    n1129 = Concatenate Strings("0101W82", w2968) -> (w2967:string)
                    n1130 = String To Byte Array(string=w2967) -> (unsigned byte array=w2980:u8[])
                    n1131 = Add Array Elements(numeric array=w2980) -> (sum=w2971:u8)
                    n1132 = Less?(x=w2971, y=u8 100) -> (x < y?=w2978:bool)
                    n1133 = case shown="False" w2978 {
                      tunnel: w2971 -> [w2985 w3072]
                      tunnel: [w2984 w3071] -> w2976
                      frame False {
                        n1134 = Quotient & Remainder(x=w2985, y=u8 10) -> (x-y*floor(x/y)=w2983:u8, floor(x/y)=w2986:u8)
                        n1135 = Subtract(x=w2986, y=u8 9) -> (x-y=w2988:u8)
                        n1136 = Number To Decimal String(number=w2983) -> (decimal integer string=w2989:string)  [unwired: 1 in]
                        n1137 = case shown="7" w2988 {
                          tunnel: w2989 -> [w2991 w2994 w2997 w3000 w3003 w3006 w3009 w3012 w3015 w3018 w3021 w3024 w3027 w3030 w3033 w3036 w3039 w3042 w3045 w3048 w3051 w3054 w3057 w3060 w3063 w3066 w3069]
                          tunnel: [w2990 w2993 w2996 w2999 w3002 w3005 w3008 w3011 w3014 w3017 w3020 w3023 w3026 w3029 w3032 w3035 w3038 w3041 w3044 w3047 w3050 w3053 w3056 w3059 w3062 w3065 w3068] -> w2984
                          frame 0, Default {
                            n1138 = Concatenate Strings("0", w2991) -> (w2990:string)
                          }
                          frame 1 {
                            n1139 = Concatenate Strings("A", w2994) -> (w2993:string)
                          }
                          frame 2 {
                            n1140 = Concatenate Strings("B", w2997) -> (w2996:string)
                          }
                          frame 3 {
                            n1141 = Concatenate Strings("C", w3000) -> (w2999:string)
                          }
                          frame 4 {
                            n1142 = Concatenate Strings("D", w3003) -> (w3002:string)
                          }
                          frame 5 {
                            n1143 = Concatenate Strings("E", w3006) -> (w3005:string)
                          }
                          frame 6 {
                            n1144 = Concatenate Strings("F", w3009) -> (w3008:string)
                          }
                          frame 7 {
                            n1145 = Concatenate Strings("G", w3012) -> (w3011:string)
                          }
                          frame 8 {
                            n1146 = Concatenate Strings("H", w3015) -> (w3014:string)
                          }
                          frame 9 {
                            n1147 = Concatenate Strings("I", w3018) -> (w3017:string)
                          }
                          frame 10 {
                            n1148 = Concatenate Strings("J", w3021) -> (w3020:string)
                          }
                          frame 11 {
                            n1149 = Concatenate Strings("K", w3024) -> (w3023:string)
                          }
                          frame 12 {
                            n1150 = Concatenate Strings("L", w3027) -> (w3026:string)
                          }
                          frame 13 {
                            n1151 = Concatenate Strings("M", w3030) -> (w3029:string)
                          }
                          frame 14 {
                            n1152 = Concatenate Strings("N", w3033) -> (w3032:string)
                          }
                          frame 15 {
                            n1153 = Concatenate Strings("O", w3036) -> (w3035:string)
                          }
                          frame 16 {
                            n1154 = Concatenate Strings("P", w3039) -> (w3038:string)
                          }
                          frame 17 {
                            n1155 = Concatenate Strings("Q", w3042) -> (w3041:string)
                          }
                          frame 18 {
                            n1156 = Concatenate Strings("R", w3045) -> (w3044:string)
                          }
                          frame 19 {
                            n1157 = Concatenate Strings("S", w3048) -> (w3047:string)
                          }
                          frame 20 {
                            n1158 = Concatenate Strings("T", w3051) -> (w3050:string)
                          }
                          frame 21 {
                            n1159 = Concatenate Strings("U", w3054) -> (w3053:string)
                          }
                          frame 22 {
                            n1160 = Concatenate Strings("V", w3057) -> (w3056:string)
                          }
                          frame 23 {
                            n1161 = Concatenate Strings("W", w3060) -> (w3059:string)
                          }
                          frame 24 {
                            n1162 = Concatenate Strings("X", w3063) -> (w3062:string)
                          }
                          frame 25 {
                            n1163 = Concatenate Strings("Y", w3066) -> (w3065:string)
                          }
                          frame 26 {
                            n1164 = Concatenate Strings("Z", w3069) -> (w3068:string)
                          }
                        }
                      }
                      frame True {
                        n1165 = Number To Decimal String(number=w3072) -> (decimal integer string=w3071:string)  [unwired: 1 in]
                      }
                    }
                    n1166 = Concatenate Strings("$", w2967, w2976, "\r") -> (w2981:string)
                    n1167 = VISA Write(VISA resource name=w2965, write buffer=w2981, error in (no error)=w2964) -> (VISA resource name out=w2970:refnum<visa-resource-name>, error out=w2969:errorcluster)  [unwired: 1 out]
                    n1168 = Wait Until Next ms Multiple(millisecond multiple=u32 300) -> ()  [unwired: 1 out]
                    n1169 = VISA Close(VISA resource name=w2970, error in (no error)=w2969) -> ()  [unwired: 1 out]
                  }
                }
              }
            }
          }
          frame 1 {
            # "Run Recipe Button Pressed"
            n1170 = Concatenate Strings("$0101W065.0000G2", "\r") -> (w3073:string)
            n1171 = VISA Write(VISA resource name=w3077, write buffer=w3073, error in (no error)=w3076) -> (VISA resource name out=w3079:refnum<visa-resource-name>, error out=w3078:errorcluster)  [unwired: 1 out]
            n1172 = VISA Close(VISA resource name=w3079, error in (no error)=w3078) -> ()  [unwired: 1 out]
          }
          frame 2 {
            # "Hold Recipe Button Pressed"
            n1173 = Concatenate Strings("$0101W066.0000G3", "\r") -> (w3082:string)
            n1174 = VISA Write(VISA resource name=w3085, write buffer=w3082, error in (no error)=w3086) -> (VISA resource name out=w3088:refnum<visa-resource-name>, error out=w3087:errorcluster)  [unwired: 1 out]
            n1175 = VISA Close(VISA resource name=w3088, error in (no error)=w3087) -> ()  [unwired: 1 out]
          }
          frame 3 {
            # "Cancel Recipe Button Pressed"
            n1176 = Concatenate Strings("$0101W063.0000G0", "\r") -> (w3093:string)
            n1177 = VISA Write(VISA resource name=w3092, write buffer=w3093, error in (no error)=w3091) -> (VISA resource name out=w3097:refnum<visa-resource-name>, error out=w3096:errorcluster)  [unwired: 1 out]
            n1178 = VISA Close(VISA resource name=w3097, error in (no error)=w3096) -> ()  [unwired: 1 out]
          }
          frame 4 {
            # "Quit Activated"
          }
        }
      }
    }
  }
